vi "SE5082_fieldramp.vi"(6 "Variables":T4=[{"Value"=10.0, "Variable"="dummy", "Save with Image"=FALSE}, {"Value"=-0.0001, "Variable"="HI", "Save with Image"=FALSE}, {"Value"=-0.0002, "Variable"="LO", "Save with Image"=FALSE}, {"Value"=0.0, "Variable"="dummy1", "Save with Image"=FALSE}, {"Value"=0.0, "Variable"="dummy2", "Save with Image"=FALSE}, {"Value"=0.0, "Variable"="dummy3", "Save with Image"=FALSE}, {"Value"=0.0, "Variable"="tLEDuv", "Save with Image"=FALSE}, {"Value"=1000.0, "Variable"="tMOT0", "Save with Image"=FALSE}, {"Value"=20.0, "Variable"="tMOT1", "Save with Image"=FALSE}, {"Value"=40.0, "Variable"="tMOT2", "Save with Image"=FALSE}, {"Value"=50.0, "Variable"="tMOT3", "Save with Image"=FALSE}, {"Value"=13.0, "Variable"="tMOT3delayREP", "Save with Image"=FALSE}, {"Value"=0.05, "Variable"="tREP", "Save with Image"=FALSE}, {"Value"=0.75, "Variable"="dMOT0", "Save with Image"=FALSE}, {"Value"=1.75, "Variable"="dMOT1", "Save with Image"=FALSE}, {"Value"=1.75, "Variable"="dMOT2", "Save with Image"=FALSE}, {"Value"=0.0, "Variable"="dummy5", "Save with Image"=FALSE}, {"Value"=1.45, "Variable"="pMOT0", "Save with Image"=FALSE}, {"Value"=1.45, "Variable"="pMOT1", "Save with Image"=FALSE}, {"Value"=1.25, "Variable"="pMOT2", "Save with Image"=FALSE}, {"Value"=-1.0, "Variable"="dummy6", "Save with Image"=FALSE}, {"Value"=1.6, "Variable"="pRP0", "Save with Image"=FALSE}, {"Value"=1.6, "Variable"="pRP1", "Save with Image"=FALSE}, {"Value"=0.8, "Variable"="pRP2", "Save with Image"=FALSE}, {"Value"=0.0, "Variable"="MOTdummy0", "Save with Image"=FALSE}, {"Value"=-1.0, "Variable"="MOTdummy1", "Save with Image"=FALSE}, {"Value"=0.0, "Variable"="MOTdummy2", "Save with Image"=FALSE}, {"Value"=0.0, "Variable"="MOTdummy3", "Save with Image"=FALSE}, {"Value"=0.0, "Variable"="MOTdummy4", "Save with Image"=FALSE}, {"Value"=1.8, "Variable"="pCROSS0", "Save with Image"=FALSE}, {"Value"=1.29, "Variable"="pCROSS1", "Save with Image"=FALSE}, {"Value"=1.05, "Variable"="pCROSS2", "Save with Image"=FALSE}, {"Value"=0.75, "Variable"="pCROSS3", "Save with Image"=FALSE}, {"Value"=0.0, "Variable"="pCROSS4", "Save with Image"=FALSE}, {"Value"=5.0, "Variable"="pDIMPL0", "Save with Image"=FALSE}, {"Value"=4.4, "Variable"="pDIMPL1", "Save with Image"=FALSE}, {"Value"=3.65, "Variable"="pDIMPL2", "Save with Image"=FALSE}, {"Value"=3.55, "Variable"="pDIMPL3", "Save with Image"=FALSE}, {"Value"=3.45, "Variable"="pDIMPL4", "Save with Image"=FALSE}, {"Value"=1.8, "Variable"="pTightTrap", "Save with Image"=FALSE}, {"Value"=400.0, "Variable"="tHOLD", "Save with Image"=FALSE}, {"Value"=740.0, "Variable"="tEVAP1", "Save with Image"=FALSE}, {"Value"=2900.0, "Variable"="tEVAP2", "Save with Image"=FALSE}, {"Value"=590.0, "Variable"="tEVAP3", "Save with Image"=FALSE}, {"Value"=50.0, "Variable"="tEVAP4", "Save with Image"=FALSE}, {"Value"=50.0, "Variable"="tHOLDTight", "Save with Image"=FALSE}, {"Value"=0.0, "Variable"="ODTdummy1", "Save with Image"=FALSE}, {"Value"=0.0, "Variable"="ODTdummy2", "Save with Image"=FALSE}, {"Value"=0.0, "Variable"="ODTdummy3", "Save with Image"=FALSE}, {"Value"=0.0, "Variable"="ODTdummy4", "Save with Image"=FALSE}, {"Value"=0.0, "Variable"="ODTdummy5", "Save with Image"=FALSE}, {"Value"=3.59, "Variable"="dIMGx", "Save with Image"=FALSE}, {"Value"=3.59, "Variable"="dIMGx0", "Save with Image"=FALSE}, {"Value"=1.38, "Variable"="dIMGz", "Save with Image"=FALSE}, {"Value"=1.98, "Variable"="dEXCz", "Save with Image"=FALSE}, {"Value"=3.0, "Variable"="pABSx", "Save with Image"=FALSE}, {"Value"=1.35, "Variable"="pABSz", "Save with Image"=FALSE}, {"Value"=0.55, "Variable"="pEXCz", "Save with Image"=FALSE}, {"Value"=0.0, "Variable"="TOF", "Save with Image"=FALSE}, {"Value"=10.0, "Variable"="TOFatomFall", "Save with Image"=FALSE}, {"Value"=0.012, "Variable"="tEXP", "Save with Image"=FALSE}, {"Value"=0.2, "Variable"="tEXP2", "Save with Image"=FALSE}, {"Value"=0.082, "Variable"="tEXC", "Save with Image"=FALSE}, {"Value"=0.001, "Variable"="tWaitIoniz", "Save with Image"=FALSE}, {"Value"=0.065, "Variable"="tCAM", "Save with Image"=FALSE}, {"Value"=200.0, "Variable"="tCAMguppy", "Save with Image"=FALSE}, {"Value"=50.0, "Variable"="tCAMreadout", "Save with Image"=FALSE}, {"Value"=-0.002, "Variable"="tTrigDelay", "Save with Image"=FALSE}, {"Value"=0.0, "Variable"="tTrans", "Save with Image"=FALSE}, {"Value"=1.0, "Variable"="tEXCres", "Save with Image"=FALSE}, {"Value"=0.004, "Variable"="tPUMP", "Save with Image"=FALSE}, {"Value"=2.0, "Variable"="pBLUEswitch", "Save with Image"=FALSE}, {"Value"=2.0, "Variable"="pBLUEswitchEIT", "Save with Image"=FALSE}, {"Value"=3.5, "Variable"="dBLUE", "Save with Image"=FALSE}, {"Value"=3.5, "Variable"="dBLUE0", "Save with Image"=FALSE}, {"Value"=1.7, "Variable"="dBLUEdec", "Save with Image"=FALSE}, {"Value"=2.5, "Variable"="dBLUEdec0", "Save with Image"=FALSE}, {"Value"=3.2, "Variable"="dIMPnew", "Save with Image"=FALSE}, {"Value"=1.0, "Variable"="blueON1", "Save with Image"=FALSE}, {"Value"=0.0, "Variable"="blueON2", "Save with Image"=FALSE}, {"Value"=1.0, "Variable"="blueEXCON1", "Save with Image"=FALSE}, {"Value"=0.0, "Variable"="blueEXCON2", "Save with Image"=FALSE}, {"Value"=35.637858, "Variable"="dRydMW", "Save with Image"=FALSE}, {"Value"=16.0, "Variable"="pRydMW", "Save with Image"=FALSE}, {"Value"=50.0, "Variable"="MWduration", "Save with Image"=FALSE}, {"Value"=4.33, "Variable"="bmw0", "Save with Image"=FALSE}, {"Value"=0.02, "Variable"="bmw1", "Save with Image"=FALSE}, {"Value"=0.0, "Variable"="MWdummy1", "Save with Image"=FALSE}, {"Value"=0.0, "Variable"="MWdummy2", "Save with Image"=FALSE}, {"Value"=0.0, "Variable"="MWdummy3", "Save with Image"=FALSE}, {"Value"=4.3, "Variable"="foffset", "Save with Image"=FALSE}, {"Value"=8.64, "Variable"="fdx", "Save with Image"=FALSE}, {"Value"=-5.78, "Variable"="fdy", "Save with Image"=FALSE}, {"Value"=4.0, "Variable"="fdz", "Save with Image"=FALSE}, {"Value"=300.0, "Variable"="CH203", "Save with Image"=FALSE}, {"Value"=160.0, "Variable"="CH215", "Save with Image"=FALSE}, {"Value"=4.0, "Variable"="CH302", "Save with Image"=FALSE}, {"Value"=280.0, "Variable"="CH315", "Save with Image"=FALSE}, {"Value"=0.0, "Variable"="CH202", "Save with Image"=FALSE}, {"Value"=0.0, "Variable"="CH308", "Save with Image"=FALSE}, {"Value"=0.0, "Variable"="EFIELDdummy2", "Save with Image"=FALSE}, {"Value"=0.0, "Variable"="EFIELDdummy3", "Save with Image"=FALSE}, {"Value"=0.0, "Variable"="EFIELDdummy4", "Save with Image"=FALSE}, {"Value"=0.0, "Variable"="EFIELDdummy5", "Save with Image"=FALSE}, {"Value"=0.0, "Variable"="EFIELDdummy6", "Save with Image"=FALSE}, {"Value"=0.0, "Variable"="EFIELDdummy7", "Save with Image"=FALSE}, {"Value"=1.25, "Variable"="bMOT0", "Save with Image"=FALSE}, {"Value"=2.5, "Variable"="bMOT1", "Save with Image"=FALSE}, {"Value"=2.5, "Variable"="bMOT2", "Save with Image"=FALSE}, {"Value"=1.25, "Variable"="bMOT3", "Save with Image"=FALSE}, {"Value"=0.0, "Variable"="bCOMPx", "Save with Image"=FALSE}, {"Value"=1.35, "Variable"="bCOMPy", "Save with Image"=FALSE}, {"Value"=0.27, "Variable"="bCOMPz", "Save with Image"=FALSE}, {"Value"=0.7, "Variable"="bCOMPx1", "Save with Image"=FALSE}, {"Value"=1.1, "Variable"="bCOMPy1", "Save with Image"=FALSE}, {"Value"=0.5, "Variable"="bCOMPz1", "Save with Image"=FALSE}, {"Value"=4.35, "Variable"="bxfinal", "Save with Image"=FALSE}, {"Value"=0.0, "Variable"="byfinal", "Save with Image"=FALSE}, {"Value"=0.0, "Variable"="bzfinal", "Save with Image"=FALSE}, {"Value"=0.0, "Variable"="BFIELDdummy1", "Save with Image"=FALSE}, {"Value"=0.0, "Variable"="BFIELDdummy2", "Save with Image"=FALSE}, {"Value"=0.0, "Variable"="BFIELDdummy3", "Save with Image"=FALSE}, {"Value"=10.0, "Variable"="tCOILsettle", "Save with Image"=FALSE}, {"Value"=0.0, "Variable"="tRemove", "Save with Image"=FALSE}, {"Value"=3.6, "Variable"="pRemove", "Save with Image"=FALSE}, {"Value"=3.1, "Variable"="dF2CLEAN1x", "Save with Image"=FALSE}, {"Value"=20.0, "Variable"="tF2CLEAN1x", "Save with Image"=FALSE}, {"Value"=4.0, "Variable"="tF2CLEAN2x", "Save with Image"=FALSE}, {"Value"=0.0, "Variable"="tDelayDown", "Save with Image"=FALSE}, {"Value"=156.0, "Variable"="oDDSbluePro", "Save with Image"=FALSE}, {"Value"=-10.25, "Variable"="dDDSbluePro", "Save with Image"=FALSE}, {"Value"=50.0, "Variable"="tRampDDSbluePro", "Save with Image"=FALSE}, {"Value"=416.6261, "Variable"="oDDSred", "Save with Image"=FALSE}, {"Value"=-50.25, "Variable"="dDDSred", "Save with Image"=FALSE}, {"Value"=90.0, "Variable"="tRampDDSred", "Save with Image"=FALSE}, {"Value"=154.0, "Variable"="oDDSblueOld", "Save with Image"=FALSE}, {"Value"=10.0, "Variable"="dDDSblueOld", "Save with Image"=FALSE}, {"Value"=100.0, "Variable"="tRampDDSblueOld", "Save with Image"=FALSE}, {"Value"=1.0, "Variable"="mwON", "Save with Image"=FALSE}, {"Value"=9.4e-05, "Variable"="tRabi", "Save with Image"=FALSE}, {"Value"=9.4e-05, "Variable"="tRabi2", "Save with Image"=FALSE}, {"Value"=5e-05, "Variable"="tRamsey", "Save with Image"=FALSE}, {"Value"=0.0, "Variable"="tRamsey2", "Save with Image"=FALSE}, {"Value"=0.0, "Variable"="tDDSa", "Save with Image"=FALSE}, {"Value"=0.0, "Variable"="tDDSb", "Save with Image"=FALSE}, {"Value"=399.942, "Variable"="dDDSa", "Save with Image"=FALSE}, {"Value"=399.942, "Variable"="dDDSa2", "Save with Image"=FALSE}, {"Value"=0.2, "Variable"="pDDSa", "Save with Image"=FALSE}, {"Value"=1e-07, "Variable"="pDDSa2", "Save with Image"=FALSE}, {"Value"=0.0, "Variable"="phiDDSa", "Save with Image"=FALSE}, {"Value"=0.875, "Variable"="phiDDSa2", "Save with Image"=FALSE}, {"Value"=399.942, "Variable"="dDDSb", "Save with Image"=FALSE}, {"Value"=400.009, "Variable"="dDDSb2", "Save with Image"=FALSE}, {"Value"=0.25, "Variable"="pDDSb", "Save with Image"=FALSE}, {"Value"=1e-07, "Variable"="pDDSb2", "Save with Image"=FALSE}, {"Value"=0.25, "Variable"="phiDDSb", "Save with Image"=FALSE}, {"Value"=0.55, "Variable"="phiDDSb2", "Save with Image"=FALSE}, {"Value"=300.0, "Variable"="tDipole", "Save with Image"=FALSE}, {"Value"=0.7, "Variable"="bCOMPx2", "Save with Image"=FALSE}, {"Value"=0.8, "Variable"="bCOMPy2", "Save with Image"=FALSE}, {"Value"=0.6, "Variable"="bCOMPz2", "Save with Image"=FALSE}, {"Value"=20.0, "Variable"="dMOTRamp1", "Save with Image"=FALSE}, {"Value"=18.0, "Variable"="DMOTload", "Save with Image"=FALSE}, {"Value"=50.0, "Variable"="dMOTRamp2", "Save with Image"=FALSE}, {"Value"=272.0, "Variable"="DMOTimag", "Save with Image"=FALSE}, {"Value"=1000.0, "Variable"="oDDShyperfine", "Save with Image"=FALSE}, {"Value"=0.1, "Variable"="dDDShyperfine", "Save with Image"=FALSE}, {"Value"=0.0, "Variable"="tof", "Save with Image"=FALSE}, {"Value"=262.5, "Variable"="dOPump", "Save with Image"=FALSE}, {"Value"=4500.0, "Variable"="tRampOPump", "Save with Image"=FALSE}, {"Value"=10.0, "Variable"="tOPump", "Save with Image"=FALSE}, {"Value"=1.5, "Variable"="bCOMPx3", "Save with Image"=FALSE}, {"Value"=0.8, "Variable"="bCOMPy3", "Save with Image"=FALSE}, {"Value"=0.0, "Variable"="bCOMPz3", "Save with Image"=FALSE}, {"Value"=0.0, "Variable"="bCOMPx4", "Save with Image"=FALSE}, {"Value"=0.0, "Variable"="bCOMPy4", "Save with Image"=FALSE}, {"Value"=0.0, "Variable"="bCOMPz4", "Save with Image"=FALSE}, {"Value"=0.0, "Variable"="scan2photRes", "Save with Image"=FALSE}, {"Value"=0.0, "Variable"="tEXCsmallProbe", "Save with Image"=FALSE}, {"Value"=0.082, "Variable"="tEXCBlue", "Save with Image"=FALSE}, {"Value"=0.0015, "Variable"="tDownPump", "Save with Image"=FALSE}, {"Value"=98.75, "Variable"="RF1freq1", "Save with Image"=FALSE}, {"Value"=0.1, "Variable"="RF1freq2", "Save with Image"=FALSE}, {"Value"=98.75, "Variable"="dummya", "Save with Image"=FALSE}, {"Value"=0.1, "Variable"="dummyb", "Save with Image"=FALSE}] {"Value" format="%#.9g"}, 8 "error in (no error)":errorcluster, 10 "HV_variables":T3={"Sampling rate"=50000000, "Amplifier gain"=-100.0, "Waveform"=[{"waveform"=1, "duration"="1", "e-factor"="-5", "Vinit"="0", "Vfinal"="1"}, {"waveform"=0, "duration"="1", "e-factor"="0", "Vinit"="1", "Vfinal"="1"}, {"waveform"=0, "duration"="1", "e-factor"="-5", "Vinit"="1", "Vfinal"="0"}], "Load waveform"=TRUE, "CH1_LO"="0", "CH1_HI"="400", "CH2_LO"="0", "CH2_HI"="-100"} {"Sampling rate" format="%.0p"; "Waveform"."waveform" items=["Linear Ramp", "Exp Rise", "Exp Decay"]}, 11 "VISA resource name in":refnum<visa-resource-name>="TCPIP0::10.11.1.75::inst0::INSTR") -> (0 "error out":errorcluster={"status"=TRUE, "code"=-1073807194, "source"="VISA Write in DG1022z_fieldramp.vi->HV_Amplifier_out.vi"}, 1 "Output to electrodes2":cluster{dbl[], "y":dbl[]}(graph)={[0.0, 0.02, 0.04, 0.06, 0.08, 0.09999999999999999, 0.12, 0.14, 0.16, 0.18, 0.19999999999999998, 0.22, 0.24, 0.26, 0.28, 0.3, 0.32, 0.33999999999999997, 0.36, 0.38, 0.39999999999999997, 0.42, 0.44, 0.45999999999999996, 0.48, 0.5, 0.52, 0.54, 0.56, 0.58, 0.6, 0.62, 0.64, 0.66, 0.6799999999999999, 0.7, 0.72, 0.74, 0.76, 0.78, 0.7999999999999999, 0.82, 0.84, 0.86, 0.88, 0.8999999999999999, 0.9199999999999999, 0.94, 0.96, 0.98, 1.0, 1.02, 1.04, 1.06, 1.08, 1.1, 1.1199999999999999, 1.14, 1.16, 1.18, 1.2, 1.22, 1.24, 1.26, 1.28, 1.2999999999999998, 1.32, 1.3399999999999999, 1.3599999999999999, 1.38, 1.4, 1.42, 1.44, 1.46, 1.4799999999999998, 1.5, 1.5199999999999998, 1.54, 1.5599999999999998, 1.5799999999999998, 1.5999999999999999, 1.6199999999999999, 1.64, 1.66, 1.68, 1.6999999999999997, 1.72, 1.7399999999999998, 1.76, 1.7799999999999998, 1.7999999999999998, 1.8199999999999998, 1.8399999999999999, 1.8599999999999999, 1.88, 1.9, 1.92, 1.9400000000000002, 1.96, 1.9799999999999998, 2.0, 2.0199999999999996, 2.04, 2.0599999999999996, 2.08, 2.0999999999999996, 2.12, 2.1399999999999997, 2.16, 2.1799999999999997, 2.2, 2.2199999999999998, 2.2399999999999998, 2.26, 2.28, 2.3, 2.32, 2.34, 2.36, 2.38, 2.4, 2.4199999999999995, 2.44, 2.4599999999999995, 2.48, 2.5, 2.52, 2.54, 2.56, 2.58, 2.5999999999999996, 2.62, 2.64, 2.66, 2.6799999999999997, 2.7, 2.7199999999999998, 2.74, 2.76, 2.7800000000000002, 2.8, 2.8200000000000003, 2.84, 2.86, 2.88, 2.9, 2.92, 2.94, 2.9599999999999995, 2.98, 3.0], "y"=[0.0, -9.580813208007743, -18.249891493826283, -26.093997906717924, -33.19163890015812, -39.61385005080873, -45.424907006445174, -50.682968778243165, -55.44065981571043, -59.745596689865145, -63.64086465588308, -67.16544886481294, -70.35462454007137, -73.24031002373526, -75.85138622603756, -78.21398567522392, -80.35175406067887, -82.28608688693284, -84.03634360706266, -85.62004137860504, -87.05303038115674, -88.34965245029956, -89.52288461551117, -90.584468978638, -91.54503023279702, -92.41418199787564, -93.2006230368708, -93.91222431603269, -94.55610778014061, -95.13871763132006, -95.66588482478362, -96.14288542699043, -96.57449342029285, -96.96502848255628, -97.31839921994724, -97.63814228557754, -97.92745777551737, -98.18924125643233, -98.42611274538788, -98.64044293186076, -98.83437690439604, -99.00985561937433, -99.16863532675555, -99.31230514721888, -99.4423029766166, -99.55992987691913, -99.66636309768043, -99.76266785834734, -99.84980800933376, -99.92865567855956, -100.0, -100.0, -100.0, -100.0, -100.0, -100.0, -100.0, -100.0, -100.0, -100.0, -100.0, -100.0, -100.0, -100.0, -100.0, -100.0, -100.0, -100.0, -100.0, -100.0, -100.0, -100.0, -100.0, -100.0, -100.0, -100.0, -100.0, -100.0, -100.0, -100.0, -100.0, -100.0, -100.0, -100.0, -100.0, -100.0, -100.0, -100.0, -100.0, -100.0, -100.0, -100.0, -100.0, -100.0, -100.0, -100.0, -100.0, -100.0, -100.0, -100.0, -100.0, -98.0, -96.0, -94.0, -92.0, -90.0, -88.0, -86.0, -84.0, -82.0, -80.0, -78.0, -76.0, -74.0, -72.0, -70.0, -68.0, -65.99999999999999, -64.0, -62.0, -60.0, -58.00000000000001, -56.00000000000001, -54.0, -52.0, -50.0, -48.0, -46.0, -43.99999999999999, -42.00000000000001, -40.0, -38.0, -36.0, -34.0, -31.999999999999996, -29.999999999999993, -28.000000000000004, -26.0, -24.0, -21.999999999999996, -19.999999999999996, -17.999999999999993, -16.000000000000004, -14.000000000000002, -12.0, -9.999999999999998, -7.9999999999999964, -5.999999999999995, -4.0000000000000036, -2.0000000000000018, 0.0]}, 2 "Output to electrodes1":cluster{dbl[], "y":dbl[]}(graph)={[0.0, 0.02, 0.04, 0.06, 0.08, 0.09999999999999999, 0.12, 0.14, 0.16, 0.18, 0.19999999999999998, 0.22, 0.24, 0.26, 0.28, 0.3, 0.32, 0.33999999999999997, 0.36, 0.38, 0.39999999999999997, 0.42, 0.44, 0.45999999999999996, 0.48, 0.5, 0.52, 0.54, 0.56, 0.58, 0.6, 0.62, 0.64, 0.66, 0.6799999999999999, 0.7, 0.72, 0.74, 0.76, 0.78, 0.7999999999999999, 0.82, 0.84, 0.86, 0.88, 0.8999999999999999, 0.9199999999999999, 0.94, 0.96, 0.98, 1.0, 1.02, 1.04, 1.06, 1.08, 1.1, 1.1199999999999999, 1.14, 1.16, 1.18, 1.2, 1.22, 1.24, 1.26, 1.28, 1.2999999999999998, 1.32, 1.3399999999999999, 1.3599999999999999, 1.38, 1.4, 1.42, 1.44, 1.46, 1.4799999999999998, 1.5, 1.5199999999999998, 1.54, 1.5599999999999998, 1.5799999999999998, 1.5999999999999999, 1.6199999999999999, 1.64, 1.66, 1.68, 1.6999999999999997, 1.72, 1.7399999999999998, 1.76, 1.7799999999999998, 1.7999999999999998, 1.8199999999999998, 1.8399999999999999, 1.8599999999999999, 1.88, 1.9, 1.92, 1.9400000000000002, 1.96, 1.9799999999999998, 2.0, 2.0199999999999996, 2.04, 2.0599999999999996, 2.08, 2.0999999999999996, 2.12, 2.1399999999999997, 2.16, 2.1799999999999997, 2.2, 2.2199999999999998, 2.2399999999999998, 2.26, 2.28, 2.3, 2.32, 2.34, 2.36, 2.38, 2.4, 2.4199999999999995, 2.44, 2.4599999999999995, 2.48, 2.5, 2.52, 2.54, 2.56, 2.58, 2.5999999999999996, 2.62, 2.64, 2.66, 2.6799999999999997, 2.7, 2.7199999999999998, 2.74, 2.76, 2.7800000000000002, 2.8, 2.8200000000000003, 2.84, 2.86, 2.88, 2.9, 2.92, 2.94, 2.9599999999999995, 2.98, 3.0], "y"=[0.0, -9.580813208007743, -18.249891493826283, -26.093997906717924, -33.19163890015812, -39.61385005080873, -45.424907006445174, -50.682968778243165, -55.44065981571043, -59.745596689865145, -63.64086465588308, -67.16544886481294, -70.35462454007137, -73.24031002373526, -75.85138622603756, -78.21398567522392, -80.35175406067887, -82.28608688693284, -84.03634360706266, -85.62004137860504, -87.05303038115674, -88.34965245029956, -89.52288461551117, -90.584468978638, -91.54503023279702, -92.41418199787564, -93.2006230368708, -93.91222431603269, -94.55610778014061, -95.13871763132006, -95.66588482478362, -96.14288542699043, -96.57449342029285, -96.96502848255628, -97.31839921994724, -97.63814228557754, -97.92745777551737, -98.18924125643233, -98.42611274538788, -98.64044293186076, -98.83437690439604, -99.00985561937433, -99.16863532675555, -99.31230514721888, -99.4423029766166, -99.55992987691913, -99.66636309768043, -99.76266785834734, -99.84980800933376, -99.92865567855956, -100.0, -100.0, -100.0, -100.0, -100.0, -100.0, -100.0, -100.0, -100.0, -100.0, -100.0, -100.0, -100.0, -100.0, -100.0, -100.0, -100.0, -100.0, -100.0, -100.0, -100.0, -100.0, -100.0, -100.0, -100.0, -100.0, -100.0, -100.0, -100.0, -100.0, -100.0, -100.0, -100.0, -100.0, -100.0, -100.0, -100.0, -100.0, -100.0, -100.0, -100.0, -100.0, -100.0, -100.0, -100.0, -100.0, -100.0, -100.0, -100.0, -100.0, -100.0, -98.0, -96.0, -94.0, -92.0, -90.0, -88.0, -86.0, -84.0, -82.0, -80.0, -78.0, -76.0, -74.0, -72.0, -70.0, -68.0, -65.99999999999999, -64.0, -62.0, -60.0, -58.00000000000001, -56.00000000000001, -54.0, -52.0, -50.0, -48.0, -46.0, -43.99999999999999, -42.00000000000001, -40.0, -38.0, -36.0, -34.0, -31.999999999999996, -29.999999999999993, -28.000000000000004, -26.0, -24.0, -21.999999999999996, -19.999999999999996, -17.999999999999993, -16.000000000000004, -14.000000000000002, -12.0, -9.999999999999998, -7.9999999999999964, -5.999999999999995, -4.0000000000000036, -2.0000000000000018, 0.0]}, 3 "VISA resource name out":refnum<visa-resource-name>="TCPIP0::10.11.1.75::inst0::INSTR")   [LabVIEW 2017]
uses:
  Software/Rydberg_Control/TypeDefinition/variables.ctl
  sequence_variables.ctl
panel:
  in  "Save sequence":bool
  in  "AWG sequence_variables":T1={"Sampling rate"=50000000, "Waveform"=[{"segment number"="1", "repeat"="-5", "jump flag"="0", "segment name"=0}, {"segment number"="1", "repeat"="0", "jump flag"="1", "segment name"=0}, {"segment number"="1", "repeat"="-5", "jump flag"="1", "segment name"=0}], "Load waveform"=FALSE, "CH1_LO"="0", "CH1_HI"="300", "CH2_LO"="0", "CH2_HI"="300"} {"Sampling rate" format="%.0p"; "Waveform"."segment name" items=["Linear Ramp", "Exp Rise", "Exp Decay"]}
  in  "Array":bool[](array[boolean])=[FALSE, TRUE]
  in  "waveform name":string[](array[string])=["000.RAF", "001.RAF"]
  in  "Debug array 2":string[](array[string])=["*CLS\n", "*RST\n", ":SOUR1:APPL:ARB 50E6,10,0", ":SOUR1:DATA VOLATILE,-0.000000,-0.049101,-0.095808,-0.140237,-0.182499,-0.222700,-0.260940,-0.297315,-0.331916,-0.364830,-0.396139,-0.425920,-0.454249,-0.481196,-0.506830,-0.531213,-0.554407,-0.576469,-0.597456,-0.617419,-0.636409,-0.654472,-0.671654,-0.687999,-0.703546,-0.718335,-0.732403,-0.745785,-0.758514,-0.770622,-0.782140,-0.793096,-0.803518,-0.813431,-0.822861,-0.831831,-0.840363,-0.848480,-0.856200,-0.863544,-0.870530,-0.877175,-0.883497,-0.889509,-0.895229,-0.900669,-0.905845,-0.910768,-0.915450,-0.919905,-0.924142,-0.928172,-0.932006,-0.935653,-0.939122,-0.942422,-0.945561,-0.948547,-0.951387,-0.954089,-0.956659,-0.959103,-0.961429,-0.963641,-0.965745,-0.967746,-0.969650,-0.971461,-0.973184,-0.974823,-0.976381,-0.977864,-0.979275,-0.980616,-0.981892,-0.983106,-0.984261,-0.985360,-0.986404,-0.987398,-0.988344,-0.989243,-0.990099,-0.990912,-0.991686,-0.992423,-0.993123,-0.993789,-0.994423,-0.995026,-0.995599,-0.996145,-0.996664,-0.997157,-0.997627,-0.998073,-0.998498,-0.998902,-0.999287,-0.999652,-1.000000,-1.000000,-1.000000,-1.000000,-1.000000,-1.000000,-1.000000,-1.000000,-1.000000,-1.000000,-1.000000,-1.000000,-1.000000,-1.000000,-1.000000,-1.000000,-1.000000,-1.000000,-1.000000,-1.000000,-1.000000,-1.000000,-1.000000,-1.000000,-1.000000,-1.000000,-1.000000,-1.000000,-1.000000,-1.000000,-1.000000,-1.000000,-1.000000,-1.000000,-1.000000,-1.000000,-1.000000,-1.000000,-1.000000,-1.000000,-1.000000,-1.000000,-1.000000,-1.000000,-1.000000,-1.000000,-1.000000,-1.000000,-1.000000,-1.000000,-1.000000,-0.980000,-0.960000,-0.940000,-0.920000,-0.900000,-0.880000,-0.860000,-0.840000,-0.820000,-0.800000,-0.780000,-0.760000,-0.740000,-0.720000,-0.700000,-0.680000,-0.660000,-0.640000,-0.620000,-0.600000,-0.580000,-0.560000,-0.540000,-0.520000,-0.500000,-0.480000,-0.460000,-0.440000,-0.420000,-0.400000,-0.380000,-0.360000,-0.340000,-0.320000,-0.300000,-0.280000,-0.260000,-0.240000,-0.220000,-0.200000,-0.180000,-0.160000,-0.140000,-0.120000,-0.100000,-0.080000,-0.060000,-0.040000,-0.020000,-0.000000", ":SOUR1:BURS:STAT ON", ":SOUR1:BURS:MODE TRIG", ":SOUR1:BURS:NCYC 1", ":SOUR1:BURS:TRIG:SOUR EXT", ":SOUR1:BURS ON", ":SOUR1:BURSt:IDLE FPT", ":OUTP:LOAD INF", ":OUTP1 ON"]
  in  "waveform name 2":string="000.RAF"
  out "Input waveform commands 2":string[](array[string])=["*CLS", "*RST", ":SOUR1:APPL:ARB 50000000", ":SOUR1:DATA VOLATILE,-0.000000,0.095808,0.182499,0.260940,0.331916,0.396139,0.454249,0.506830,0.554407,0.597456,0.636409,0.671654,0.703546,0.732403,0.758514,0.782140,0.803518,0.822861,0.840363,0.856200,0.870530,0.883497,0.895229,0.905845,0.915450,0.924142,0.932006,0.939122,0.945561,0.951387,0.956659,0.961429,0.965745,0.969650,0.973184,0.976381,0.979275,0.981892,0.984261,0.986404,0.988344,0.990099,0.991686,0.993123,0.994423,0.995599,0.996664,0.997627,0.998498,0.999287,1.000000,1.000000,1.000000,1.000000,1.000000,1.000000,1.000000,1.000000,1.000000,1.000000,1.000000,1.000000,1.000000,1.000000,1.000000,1.000000,1.000000,1.000000,1.000000,1.000000,1.000000,1.000000,1.000000,1.000000,1.000000,1.000000,1.000000,1.000000,1.000000,1.000000,1.000000,1.000000,1.000000,1.000000,1.000000,1.000000,1.000000,1.000000,1.000000,1.000000,1.000000,1.000000,1.000000,1.000000,1.000000,1.000000,1.000000,1.000000,1.000000,1.000000,1.000000,0.980000,0.960000,0.940000,0.920000,0.900000,0.880000,0.860000,0.840000,0.820000,0.800000,0.780000,0.760000,0.740000,0.720000,0.700000,0.680000,0.660000,0.640000,0.620000,0.600000,0.580000,0.560000,0.540000,0.520000,0.500000,0.480000,0.460000,0.440000,0.420000,0.400000,0.380000,0.360000,0.340000,0.320000,0.300000,0.280000,0.260000,0.240000,0.220000,0.200000,0.180000,0.160000,0.140000,0.120000,0.100000,0.080000,0.060000,0.040000,0.020000,-0.000000", ":SOUR1:DATA:COPY 000.RAF, VOLATILE", ":SOUR1:FUNC USER 000.RAF", ":SOUR1:BURS:STAT ON", ":SOUR1:BURS:MODE TRIG", ":SOUR1:BURS:NCYC 1", ":SOUR1:BURS:TRIG:SOUR EXT", ":SOUR1:BURS ON", ":SOUR1:BURSt:IDLE FPT", ":OUTP:LOAD INF"]
  out "waveform to CH2":dbl[](array[numeric])=[-0.0, 0.09580813208007743, 0.18249891493826284, 0.26093997906717925, 0.33191638900158116, 0.3961385005080873, 0.45424907006445175, 0.5068296877824316, 0.5544065981571044, 0.5974559668986514, 0.6364086465588308, 0.6716544886481295, 0.7035462454007138, 0.7324031002373527, 0.7585138622603756, 0.7821398567522393, 0.8035175406067887, 0.8228608688693284, 0.8403634360706266, 0.8562004137860504, 0.8705303038115675, 0.8834965245029955, 0.8952288461551118, 0.90584468978638, 0.9154503023279702, 0.9241418199787564, 0.932006230368708, 0.9391222431603269, 0.9455610778014061, 0.9513871763132006, 0.9566588482478362, 0.9614288542699043, 0.9657449342029285, 0.9696502848255628, 0.9731839921994724, 0.9763814228557754, 0.9792745777551737, 0.9818924125643232, 0.9842611274538788, 0.9864044293186076, 0.9883437690439604, 0.9900985561937433, 0.9916863532675555, 0.9931230514721888, 0.994423029766166, 0.9955992987691913, 0.9966636309768043, 0.9976266785834734, 0.9984980800933375, 0.9992865567855956, 1.0, 1.0, 1.0, 1.0, 1.0, 1.0, 1.0, 1.0, 1.0, 1.0, 1.0, 1.0, 1.0, 1.0, 1.0, 1.0, 1.0, 1.0, 1.0, 1.0, 1.0, 1.0, 1.0, 1.0, 1.0, 1.0, 1.0, 1.0, 1.0, 1.0, 1.0, 1.0, 1.0, 1.0, 1.0, 1.0, 1.0, 1.0, 1.0, 1.0, 1.0, 1.0, 1.0, 1.0, 1.0, 1.0, 1.0, 1.0, 1.0, 1.0, 1.0, 0.98, 0.96, 0.94, 0.92, 0.9, 0.88, 0.86, 0.84, 0.82, 0.8, 0.78, 0.76, 0.74, 0.72, 0.7, 0.68, 0.6599999999999998, 0.64, 0.62, 0.6, 0.5800000000000001, 0.56, 0.54, 0.52, 0.5, 0.48, 0.46, 0.43999999999999995, 0.4200000000000001, 0.4, 0.38, 0.36, 0.34, 0.31999999999999995, 0.29999999999999993, 0.28, 0.26, 0.24, 0.21999999999999997, 0.19999999999999996, 0.17999999999999994, 0.16000000000000003, 0.14, 0.12, 0.09999999999999998, 0.07999999999999996, 0.05999999999999995, 0.040000000000000036, 0.020000000000000018, -0.0]
  out "Output to CH2":dbl[](graph)=[-0.0, 0.09580813208007743, 0.18249891493826284, 0.26093997906717925, 0.33191638900158116, 0.3961385005080873, 0.45424907006445175, 0.5068296877824316, 0.5544065981571044, 0.5974559668986514, 0.6364086465588308, 0.6716544886481295, 0.7035462454007138, 0.7324031002373527, 0.7585138622603756, 0.7821398567522393, 0.8035175406067887, 0.8228608688693284, 0.8403634360706266, 0.8562004137860504, 0.8705303038115675, 0.8834965245029955, 0.8952288461551118, 0.90584468978638, 0.9154503023279702, 0.9241418199787564, 0.932006230368708, 0.9391222431603269, 0.9455610778014061, 0.9513871763132006, 0.9566588482478362, 0.9614288542699043, 0.9657449342029285, 0.9696502848255628, 0.9731839921994724, 0.9763814228557754, 0.9792745777551737, 0.9818924125643232, 0.9842611274538788, 0.9864044293186076, 0.9883437690439604, 0.9900985561937433, 0.9916863532675555, 0.9931230514721888, 0.994423029766166, 0.9955992987691913, 0.9966636309768043, 0.9976266785834734, 0.9984980800933375, 0.9992865567855956, 1.0, 1.0, 1.0, 1.0, 1.0, 1.0, 1.0, 1.0, 1.0, 1.0, 1.0, 1.0, 1.0, 1.0, 1.0, 1.0, 1.0, 1.0, 1.0, 1.0, 1.0, 1.0, 1.0, 1.0, 1.0, 1.0, 1.0, 1.0, 1.0, 1.0, 1.0, 1.0, 1.0, 1.0, 1.0, 1.0, 1.0, 1.0, 1.0, 1.0, 1.0, 1.0, 1.0, 1.0, 1.0, 1.0, 1.0, 1.0, 1.0, 1.0, 1.0, 0.98, 0.96, 0.94, 0.92, 0.9, 0.88, 0.86, 0.84, 0.82, 0.8, 0.78, 0.76, 0.74, 0.72, 0.7, 0.68, 0.6599999999999998, 0.64, 0.62, 0.6, 0.5800000000000001, 0.56, 0.54, 0.52, 0.5, 0.48, 0.46, 0.43999999999999995, 0.4200000000000001, 0.4, 0.38, 0.36, 0.34, 0.31999999999999995, 0.29999999999999993, 0.28, 0.26, 0.24, 0.21999999999999997, 0.19999999999999996, 0.17999999999999994, 0.16000000000000003, 0.14, 0.12, 0.09999999999999998, 0.07999999999999996, 0.05999999999999995, 0.040000000000000036, 0.020000000000000018, -0.0]
  out "hvhi2":dbl
  out "hvlo2":dbl
  out "CH2_LO":string="0"
  out "CH2_HI":string="-100"
  out "hvlo1":dbl
  out "hvhi1":dbl
  in  "Readout status?":bool
  out "Load waveform":bool=TRUE
  out "Amplifier gain":dbl=-100.0
  out "CH1_HI":string="-100"
  out "CH1_LO":string="0"
  out "Sampling rate":i32=50000000 format="%.0p"
  out "Waveform":T2(array[cluster])=[{"waveform"=1, "duration"="1", "e-factor"="-5", "Vinit"="0", "Vfinal"="1"}, {"waveform"=0, "duration"="1", "e-factor"="0", "Vinit"="1", "Vfinal"="1"}, {"waveform"=0, "duration"="1", "e-factor"="-5", "Vinit"="1", "Vfinal"="0"}]
  out "Input waveform commands":string[](array[string])=["*CLS", "*RST", ":SOUR1:APPL:ARB 50000000", ":SOUR1:DATA VOLATILE,-0.000000,0.095808,0.182499,0.260940,0.331916,0.396139,0.454249,0.506830,0.554407,0.597456,0.636409,0.671654,0.703546,0.732403,0.758514,0.782140,0.803518,0.822861,0.840363,0.856200,0.870530,0.883497,0.895229,0.905845,0.915450,0.924142,0.932006,0.939122,0.945561,0.951387,0.956659,0.961429,0.965745,0.969650,0.973184,0.976381,0.979275,0.981892,0.984261,0.986404,0.988344,0.990099,0.991686,0.993123,0.994423,0.995599,0.996664,0.997627,0.998498,0.999287,1.000000,1.000000,1.000000,1.000000,1.000000,1.000000,1.000000,1.000000,1.000000,1.000000,1.000000,1.000000,1.000000,1.000000,1.000000,1.000000,1.000000,1.000000,1.000000,1.000000,1.000000,1.000000,1.000000,1.000000,1.000000,1.000000,1.000000,1.000000,1.000000,1.000000,1.000000,1.000000,1.000000,1.000000,1.000000,1.000000,1.000000,1.000000,1.000000,1.000000,1.000000,1.000000,1.000000,1.000000,1.000000,1.000000,1.000000,1.000000,1.000000,1.000000,1.000000,0.980000,0.960000,0.940000,0.920000,0.900000,0.880000,0.860000,0.840000,0.820000,0.800000,0.780000,0.760000,0.740000,0.720000,0.700000,0.680000,0.660000,0.640000,0.620000,0.600000,0.580000,0.560000,0.540000,0.520000,0.500000,0.480000,0.460000,0.440000,0.420000,0.400000,0.380000,0.360000,0.340000,0.320000,0.300000,0.280000,0.260000,0.240000,0.220000,0.200000,0.180000,0.160000,0.140000,0.120000,0.100000,0.080000,0.060000,0.040000,0.020000,-0.000000", ":SOUR1:DATA:COPY 000.RAF, VOLATILE", ":SOUR1:FUNC USER 000.RAF", ":SOUR1:BURS:STAT ON", ":SOUR1:BURS:MODE TRIG", ":SOUR1:BURS:NCYC 1", ":SOUR1:BURS:TRIG:SOUR EXT", ":SOUR1:BURS ON", ":SOUR1:BURSt:IDLE FPT", ":OUTP:LOAD INF"]
  in  "Read-out commands":string[](array[string])=["*IDN?", ":SOUR1:APPL?", ":SOUR1:BURS:STAT?", ":SOUR1:BURS:TRIG:SOUR?", ":OUTP1:LOAD?", ":SOUR2:APPL?", ":SOUR2:BURS:STAT?", ":SOUR2:BURS:TRIG:SOUR?", ":OUTP2:LOAD?", ":SOUR2:FUNC?"]
  out "Output to CH1":dbl[](graph)=[-0.0, 0.09580813208007743, 0.18249891493826284, 0.26093997906717925, 0.33191638900158116, 0.3961385005080873, 0.45424907006445175, 0.5068296877824316, 0.5544065981571044, 0.5974559668986514, 0.6364086465588308, 0.6716544886481295, 0.7035462454007138, 0.7324031002373527, 0.7585138622603756, 0.7821398567522393, 0.8035175406067887, 0.8228608688693284, 0.8403634360706266, 0.8562004137860504, 0.8705303038115675, 0.8834965245029955, 0.8952288461551118, 0.90584468978638, 0.9154503023279702, 0.9241418199787564, 0.932006230368708, 0.9391222431603269, 0.9455610778014061, 0.9513871763132006, 0.9566588482478362, 0.9614288542699043, 0.9657449342029285, 0.9696502848255628, 0.9731839921994724, 0.9763814228557754, 0.9792745777551737, 0.9818924125643232, 0.9842611274538788, 0.9864044293186076, 0.9883437690439604, 0.9900985561937433, 0.9916863532675555, 0.9931230514721888, 0.994423029766166, 0.9955992987691913, 0.9966636309768043, 0.9976266785834734, 0.9984980800933375, 0.9992865567855956, 1.0, 1.0, 1.0, 1.0, 1.0, 1.0, 1.0, 1.0, 1.0, 1.0, 1.0, 1.0, 1.0, 1.0, 1.0, 1.0, 1.0, 1.0, 1.0, 1.0, 1.0, 1.0, 1.0, 1.0, 1.0, 1.0, 1.0, 1.0, 1.0, 1.0, 1.0, 1.0, 1.0, 1.0, 1.0, 1.0, 1.0, 1.0, 1.0, 1.0, 1.0, 1.0, 1.0, 1.0, 1.0, 1.0, 1.0, 1.0, 1.0, 1.0, 1.0, 0.98, 0.96, 0.94, 0.92, 0.9, 0.88, 0.86, 0.84, 0.82, 0.8, 0.78, 0.76, 0.74, 0.72, 0.7, 0.68, 0.6599999999999998, 0.64, 0.62, 0.6, 0.5800000000000001, 0.56, 0.54, 0.52, 0.5, 0.48, 0.46, 0.43999999999999995, 0.4200000000000001, 0.4, 0.38, 0.36, 0.34, 0.31999999999999995, 0.29999999999999993, 0.28, 0.26, 0.24, 0.21999999999999997, 0.19999999999999996, 0.17999999999999994, 0.16000000000000003, 0.14, 0.12, 0.09999999999999998, 0.07999999999999996, 0.05999999999999995, 0.040000000000000036, 0.020000000000000018, -0.0]
  out "Status output":string[](array[string])
  out "waveform to CH1":dbl[](array[numeric])=[-0.0, 0.09580813208007743, 0.18249891493826284, 0.26093997906717925, 0.33191638900158116, 0.3961385005080873, 0.45424907006445175, 0.5068296877824316, 0.5544065981571044, 0.5974559668986514, 0.6364086465588308, 0.6716544886481295, 0.7035462454007138, 0.7324031002373527, 0.7585138622603756, 0.7821398567522393, 0.8035175406067887, 0.8228608688693284, 0.8403634360706266, 0.8562004137860504, 0.8705303038115675, 0.8834965245029955, 0.8952288461551118, 0.90584468978638, 0.9154503023279702, 0.9241418199787564, 0.932006230368708, 0.9391222431603269, 0.9455610778014061, 0.9513871763132006, 0.9566588482478362, 0.9614288542699043, 0.9657449342029285, 0.9696502848255628, 0.9731839921994724, 0.9763814228557754, 0.9792745777551737, 0.9818924125643232, 0.9842611274538788, 0.9864044293186076, 0.9883437690439604, 0.9900985561937433, 0.9916863532675555, 0.9931230514721888, 0.994423029766166, 0.9955992987691913, 0.9966636309768043, 0.9976266785834734, 0.9984980800933375, 0.9992865567855956, 1.0, 1.0, 1.0, 1.0, 1.0, 1.0, 1.0, 1.0, 1.0, 1.0, 1.0, 1.0, 1.0, 1.0, 1.0, 1.0, 1.0, 1.0, 1.0, 1.0, 1.0, 1.0, 1.0, 1.0, 1.0, 1.0, 1.0, 1.0, 1.0, 1.0, 1.0, 1.0, 1.0, 1.0, 1.0, 1.0, 1.0, 1.0, 1.0, 1.0, 1.0, 1.0, 1.0, 1.0, 1.0, 1.0, 1.0, 1.0, 1.0, 1.0, 1.0, 0.98, 0.96, 0.94, 0.92, 0.9, 0.88, 0.86, 0.84, 0.82, 0.8, 0.78, 0.76, 0.74, 0.72, 0.7, 0.68, 0.6599999999999998, 0.64, 0.62, 0.6, 0.5800000000000001, 0.56, 0.54, 0.52, 0.5, 0.48, 0.46, 0.43999999999999995, 0.4200000000000001, 0.4, 0.38, 0.36, 0.34, 0.31999999999999995, 0.29999999999999993, 0.28, 0.26, 0.24, 0.21999999999999997, 0.19999999999999996, 0.17999999999999994, 0.16000000000000003, 0.14, 0.12, 0.09999999999999998, 0.07999999999999996, 0.05999999999999995, 0.040000000000000036, 0.020000000000000018, -0.0]
  out "Plot X":dbl[](graph)=[0.0, 2e-08, 4e-08, 6e-08, 8e-08, 1e-07, 1.2e-07, 1.4e-07, 1.6e-07, 1.8e-07, 2e-07, 2.2e-07, 2.4e-07, 2.6e-07, 2.8e-07, 3e-07, 3.2e-07, 3.4e-07, 3.6e-07, 3.8e-07, 4e-07, 4.2e-07, 4.4e-07, 4.6e-07, 4.8e-07, 5e-07, 5.2e-07, 5.4e-07, 5.6e-07, 5.8e-07, 6e-07, 6.2e-07, 6.4e-07, 6.6e-07, 6.8e-07, 7e-07, 7.2e-07, 7.4e-07, 7.6e-07, 7.8e-07, 8e-07, 8.2e-07, 8.4e-07, 8.6e-07, 8.8e-07, 9e-07, 9.2e-07, 9.4e-07, 9.6e-07, 9.8e-07, 1e-06, 1.02e-06, 1.04e-06, 1.06e-06, 1.08e-06, 1.1e-06, 1.1199999999999999e-06, 1.1399999999999999e-06, 1.16e-06, 1.18e-06, 1.2e-06, 1.22e-06, 1.24e-06, 1.26e-06, 1.28e-06, 1.2999999999999998e-06, 1.32e-06, 1.3399999999999999e-06, 1.36e-06, 1.38e-06, 1.4e-06, 1.42e-06, 1.44e-06, 1.46e-06, 1.4799999999999998e-06, 1.5e-06, 1.5199999999999998e-06, 1.54e-06, 1.5599999999999999e-06, 1.58e-06, 1.6e-06, 1.62e-06, 1.64e-06, 1.66e-06, 1.68e-06, 1.6999999999999998e-06, 1.72e-06, 1.7399999999999999e-06, 1.76e-06, 1.78e-06, 1.8e-06, 1.82e-06, 1.84e-06, 1.86e-06, 1.88e-06, 1.9e-06, 1.92e-06, 1.94e-06, 1.96e-06, 1.9799999999999997e-06, 2e-06, 2.0199999999999997e-06, 2.04e-06, 2.0599999999999998e-06, 2.08e-06, 2.1e-06, 2.12e-06, 2.14e-06, 2.16e-06, 2.18e-06, 2.2e-06, 2.22e-06, 2.2399999999999997e-06, 2.26e-06, 2.2799999999999998e-06, 2.3e-06, 2.32e-06, 2.34e-06, 2.36e-06, 2.38e-06, 2.4e-06, 2.4199999999999997e-06, 2.44e-06, 2.4599999999999997e-06, 2.48e-06, 2.4999999999999998e-06, 2.52e-06, 2.54e-06, 2.56e-06, 2.58e-06, 2.5999999999999997e-06, 2.62e-06, 2.64e-06, 2.66e-06, 2.6799999999999998e-06, 2.7e-06, 2.72e-06, 2.74e-06, 2.76e-06, 2.78e-06, 2.8e-06, 2.82e-06, 2.84e-06, 2.8599999999999997e-06, 2.88e-06, 2.8999999999999998e-06, 2.92e-06, 2.94e-06, 2.9599999999999996e-06, 2.98e-06, 3e-06]
  out "x":dbl[](array[numeric])=[0.0, 2e-08, 4e-08, 6e-08, 8e-08, 1e-07, 1.2e-07, 1.4e-07, 1.6e-07, 1.8e-07, 2e-07, 2.2e-07, 2.4e-07, 2.6e-07, 2.8e-07, 3e-07, 3.2e-07, 3.4e-07, 3.6e-07, 3.8e-07, 4e-07, 4.2e-07, 4.4e-07, 4.6e-07, 4.8e-07, 5e-07, 5.2e-07, 5.4e-07, 5.6e-07, 5.8e-07, 6e-07, 6.2e-07, 6.4e-07, 6.6e-07, 6.8e-07, 7e-07, 7.2e-07, 7.4e-07, 7.6e-07, 7.8e-07, 8e-07, 8.2e-07, 8.4e-07, 8.6e-07, 8.8e-07, 9e-07, 9.2e-07, 9.4e-07, 9.6e-07, 9.8e-07, 1e-06, 1.02e-06, 1.04e-06, 1.06e-06, 1.08e-06, 1.1e-06, 1.1199999999999999e-06, 1.1399999999999999e-06, 1.16e-06, 1.18e-06, 1.2e-06, 1.22e-06, 1.24e-06, 1.26e-06, 1.28e-06, 1.2999999999999998e-06, 1.32e-06, 1.3399999999999999e-06, 1.36e-06, 1.38e-06, 1.4e-06, 1.42e-06, 1.44e-06, 1.46e-06, 1.4799999999999998e-06, 1.5e-06, 1.5199999999999998e-06, 1.54e-06, 1.5599999999999999e-06, 1.58e-06, 1.6e-06, 1.62e-06, 1.64e-06, 1.66e-06, 1.68e-06, 1.6999999999999998e-06, 1.72e-06, 1.7399999999999999e-06, 1.76e-06, 1.78e-06, 1.8e-06, 1.82e-06, 1.84e-06, 1.86e-06, 1.88e-06, 1.9e-06, 1.92e-06, 1.94e-06, 1.96e-06, 1.9799999999999997e-06, 2e-06, 2.0199999999999997e-06, 2.04e-06, 2.0599999999999998e-06, 2.08e-06, 2.1e-06, 2.12e-06, 2.14e-06, 2.16e-06, 2.18e-06, 2.2e-06, 2.22e-06, 2.2399999999999997e-06, 2.26e-06, 2.2799999999999998e-06, 2.3e-06, 2.32e-06, 2.34e-06, 2.36e-06, 2.38e-06, 2.4e-06, 2.4199999999999997e-06, 2.44e-06, 2.4599999999999997e-06, 2.48e-06, 2.4999999999999998e-06, 2.52e-06, 2.54e-06, 2.56e-06, 2.58e-06, 2.5999999999999997e-06, 2.62e-06, 2.64e-06, 2.66e-06, 2.6799999999999998e-06, 2.7e-06, 2.72e-06, 2.74e-06, 2.76e-06, 2.78e-06, 2.8e-06, 2.82e-06, 2.84e-06, 2.8599999999999997e-06, 2.88e-06, 2.8999999999999998e-06, 2.92e-06, 2.94e-06, 2.9599999999999996e-06, 2.98e-06, 3e-06]
  out "y":dbl[](array[numeric])=[0.0, 0.09580813208007743, 0.1824989149382628, 0.26093997906717925, 0.33191638900158116, 0.3961385005080873, 0.45424907006445175, 0.5068296877824316, 0.5544065981571044, 0.5974559668986514, 0.6364086465588308, 0.6716544886481295, 0.7035462454007136, 0.7324031002373527, 0.7585138622603756, 0.7821398567522392, 0.8035175406067887, 0.8228608688693284, 0.8403634360706267, 0.8562004137860504, 0.8705303038115675, 0.8834965245029955, 0.8952288461551118, 0.90584468978638, 0.9154503023279702, 0.9241418199787564, 0.932006230368708, 0.9391222431603269, 0.9455610778014061, 0.9513871763132007, 0.9566588482478362, 0.9614288542699043, 0.9657449342029285, 0.9696502848255628, 0.9731839921994724, 0.9763814228557754, 0.9792745777551737, 0.9818924125643232, 0.9842611274538788, 0.9864044293186076, 0.9883437690439604, 0.9900985561937433, 0.9916863532675555, 0.9931230514721888, 0.994423029766166, 0.9955992987691913, 0.9966636309768043, 0.9976266785834734, 0.9984980800933375, 0.9992865567855956, 1.0, 1.0, 1.0, 1.0, 1.0, 1.0, 1.0, 1.0, 1.0, 1.0, 1.0, 1.0, 1.0, 1.0, 1.0, 1.0, 1.0, 1.0, 1.0, 1.0, 1.0, 1.0, 1.0, 1.0, 1.0, 1.0, 1.0, 1.0, 1.0, 1.0, 1.0, 1.0, 1.0, 1.0, 1.0, 1.0, 1.0, 1.0, 1.0, 1.0, 1.0, 1.0, 1.0, 1.0, 1.0, 1.0, 1.0, 1.0, 1.0, 1.0, 1.0, 0.98, 0.96, 0.94, 0.92, 0.9, 0.88, 0.86, 0.84, 0.8200000000000001, 0.8, 0.78, 0.76, 0.74, 0.72, 0.7, 0.6799999999999999, 0.6599999999999999, 0.64, 0.62, 0.6, 0.5800000000000001, 0.56, 0.54, 0.52, 0.5, 0.48, 0.45999999999999996, 0.43999999999999995, 0.42000000000000004, 0.4, 0.38, 0.36, 0.33999999999999997, 0.31999999999999995, 0.29999999999999993, 0.28, 0.26, 0.24, 0.21999999999999997, 0.19999999999999996, 0.17999999999999994, 0.16000000000000003, 0.14, 0.12, 0.09999999999999998, 0.07999999999999996, 0.05999999999999994, 0.040000000000000036, 0.020000000000000018, 0.0]
  out "time for waveform":dbl[](array[numeric])=[0.0, 1e-06, 2e-06]
  out "timestep (ideal)":dbl[](array[numeric])=[1e-06, 2e-06, 3e-06]
  out "timestep":dbl[](array[numeric])=[50.0, 100.0, 150.0]
  out "timestep (int)":i32[](array[numeric])=[0, 50, 100]
  out "segment duration (int)":i32[](array[numeric])=[50, 50, 50]
  out "segment duration":dbl[](array[numeric])=[50.0, 50.0, 50.0]
  out "Plot Y":dbl[](graph)=[0.0, 0.09580813208007743, 0.1824989149382628, 0.26093997906717925, 0.33191638900158116, 0.3961385005080873, 0.45424907006445175, 0.5068296877824316, 0.5544065981571044, 0.5974559668986514, 0.6364086465588308, 0.6716544886481295, 0.7035462454007136, 0.7324031002373527, 0.7585138622603756, 0.7821398567522392, 0.8035175406067887, 0.8228608688693284, 0.8403634360706267, 0.8562004137860504, 0.8705303038115675, 0.8834965245029955, 0.8952288461551118, 0.90584468978638, 0.9154503023279702, 0.9241418199787564, 0.932006230368708, 0.9391222431603269, 0.9455610778014061, 0.9513871763132007, 0.9566588482478362, 0.9614288542699043, 0.9657449342029285, 0.9696502848255628, 0.9731839921994724, 0.9763814228557754, 0.9792745777551737, 0.9818924125643232, 0.9842611274538788, 0.9864044293186076, 0.9883437690439604, 0.9900985561937433, 0.9916863532675555, 0.9931230514721888, 0.994423029766166, 0.9955992987691913, 0.9966636309768043, 0.9976266785834734, 0.9984980800933375, 0.9992865567855956, 1.0, 1.0, 1.0, 1.0, 1.0, 1.0, 1.0, 1.0, 1.0, 1.0, 1.0, 1.0, 1.0, 1.0, 1.0, 1.0, 1.0, 1.0, 1.0, 1.0, 1.0, 1.0, 1.0, 1.0, 1.0, 1.0, 1.0, 1.0, 1.0, 1.0, 1.0, 1.0, 1.0, 1.0, 1.0, 1.0, 1.0, 1.0, 1.0, 1.0, 1.0, 1.0, 1.0, 1.0, 1.0, 1.0, 1.0, 1.0, 1.0, 1.0, 1.0, 0.98, 0.96, 0.94, 0.92, 0.9, 0.88, 0.86, 0.84, 0.8200000000000001, 0.8, 0.78, 0.76, 0.74, 0.72, 0.7, 0.6799999999999999, 0.6599999999999999, 0.64, 0.62, 0.6, 0.5800000000000001, 0.56, 0.54, 0.52, 0.5, 0.48, 0.45999999999999996, 0.43999999999999995, 0.42000000000000004, 0.4, 0.38, 0.36, 0.33999999999999997, 0.31999999999999995, 0.29999999999999993, 0.28, 0.26, 0.24, 0.21999999999999997, 0.19999999999999996, 0.17999999999999994, 0.16000000000000003, 0.14, 0.12, 0.09999999999999998, 0.07999999999999996, 0.05999999999999994, 0.040000000000000036, 0.020000000000000018, 0.0]
  # "Indicator"
  # "Commands that cause error:\n:SOUR1:DATA:COPY 000.RAF, VOLATILE\n:SOUR1:FUNC USER 000.RAF"
  # "Max 5 GSa/s"
  # "segment"
  # "segment name"
  # "repeat"
  # "jump flag"
  # "Resolution: 20ns, Range(Vint, Vfinal) is +/-1V\nIf e-factor =0 for exp rise/exp decay, will get NaN"
  # "Max 60 MSa/s\nfor arbitrary wf\nDefault: 50M"
  # "loss 5 % on a resistor"
  # "V initial"
  # "V final"
  # "Waveform"
  # "duration (us)"
  # "e-factor"
  # "Resolution: 20ns, Range(Vint, Vfinal) is +/-1V\nIf e-factor =0 for exp rise/exp decay, will get NaN"
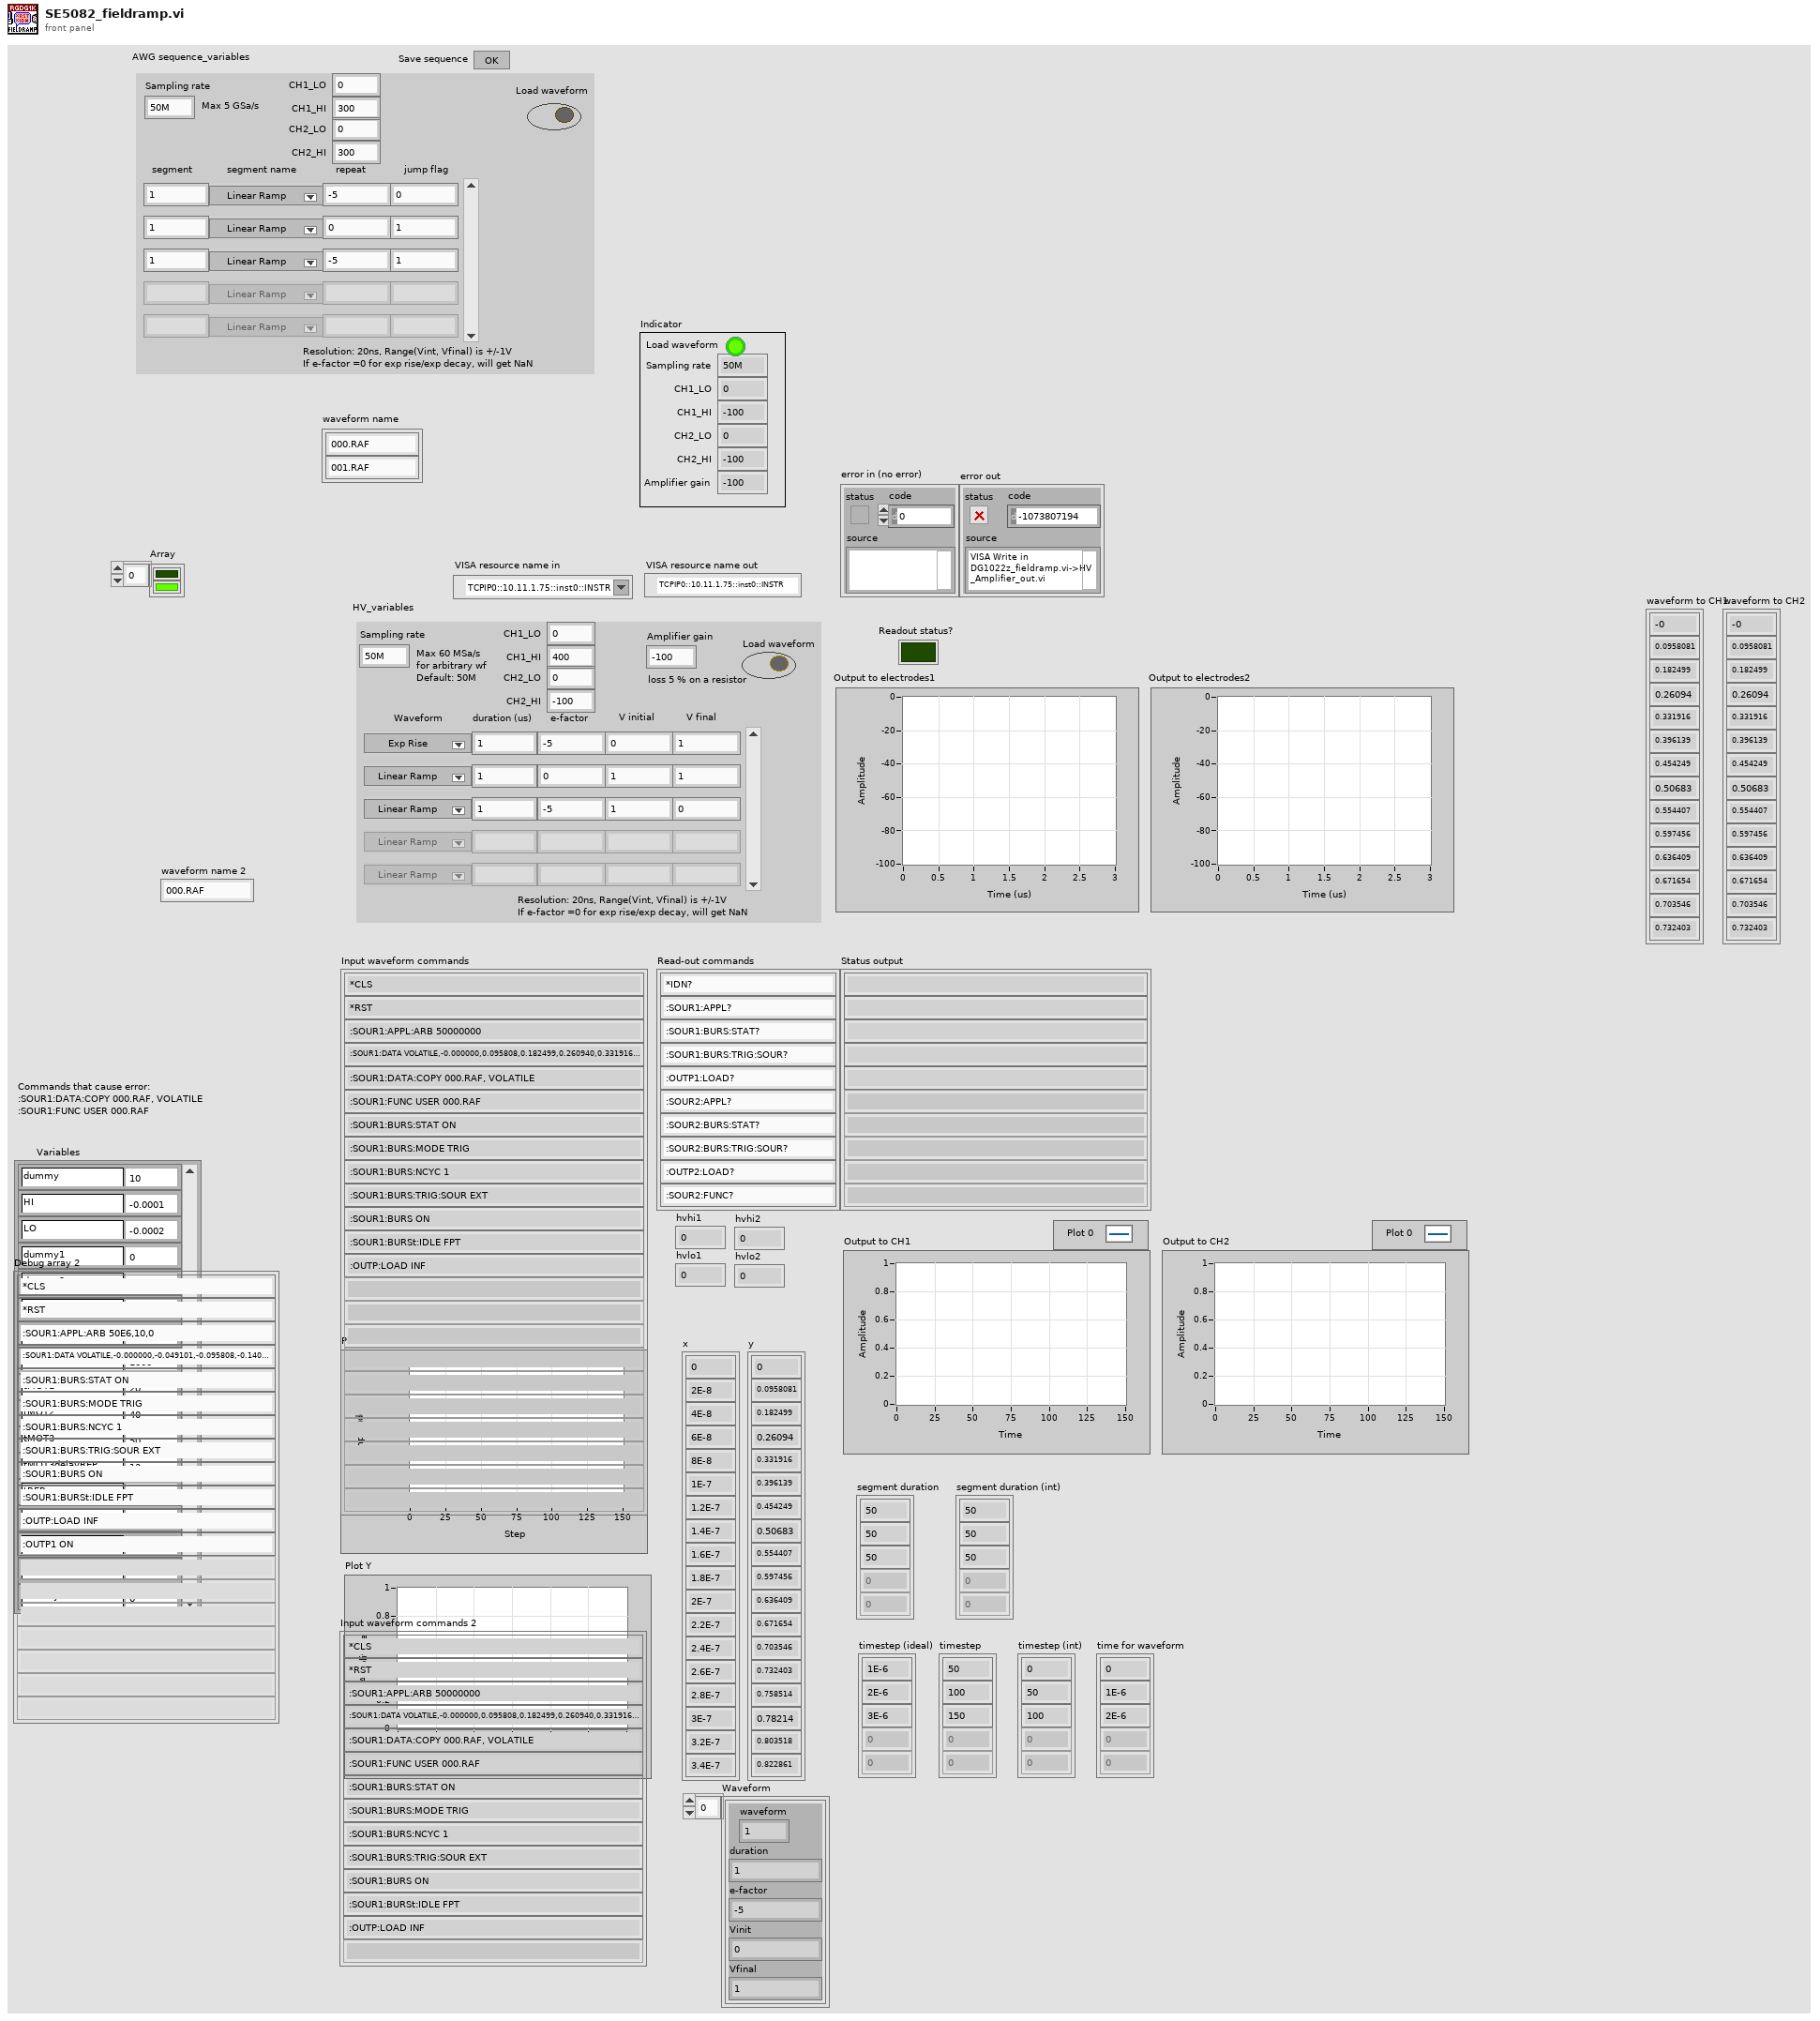
[diagram p1: front panel]
types:
  T1 = typedef "sequence_variables.ctl" = cluster{"Sampling rate":i32, "Waveform":cluster{"segment number":string, "repeat":string, "jump flag":string, "segment name":u16}[], "Load waveform":bool, "CH1_LO":string, "CH1_HI":string, "CH2_LO":string, "CH2_HI":string}
  T2 = cluster{"waveform":u16, "duration":string, "e-factor":string, "Vinit":string, "Vfinal":string}[]
  T3 = typedef "HV_variables.ctl" = cluster{"Sampling rate":i32, "Amplifier gain":dbl, "Waveform":cluster{"waveform":u16, "duration":string, "e-factor":string, "Vinit":string, "Vfinal":string}[], "Load waveform":bool, "CH1_LO":string, "CH1_HI":string, "CH2_LO":string, "CH2_HI":string}
  T4 = typedef "variables.ctl" = cluster{"Value":dbl, "Variable":string, "Save with Image":bool}[]
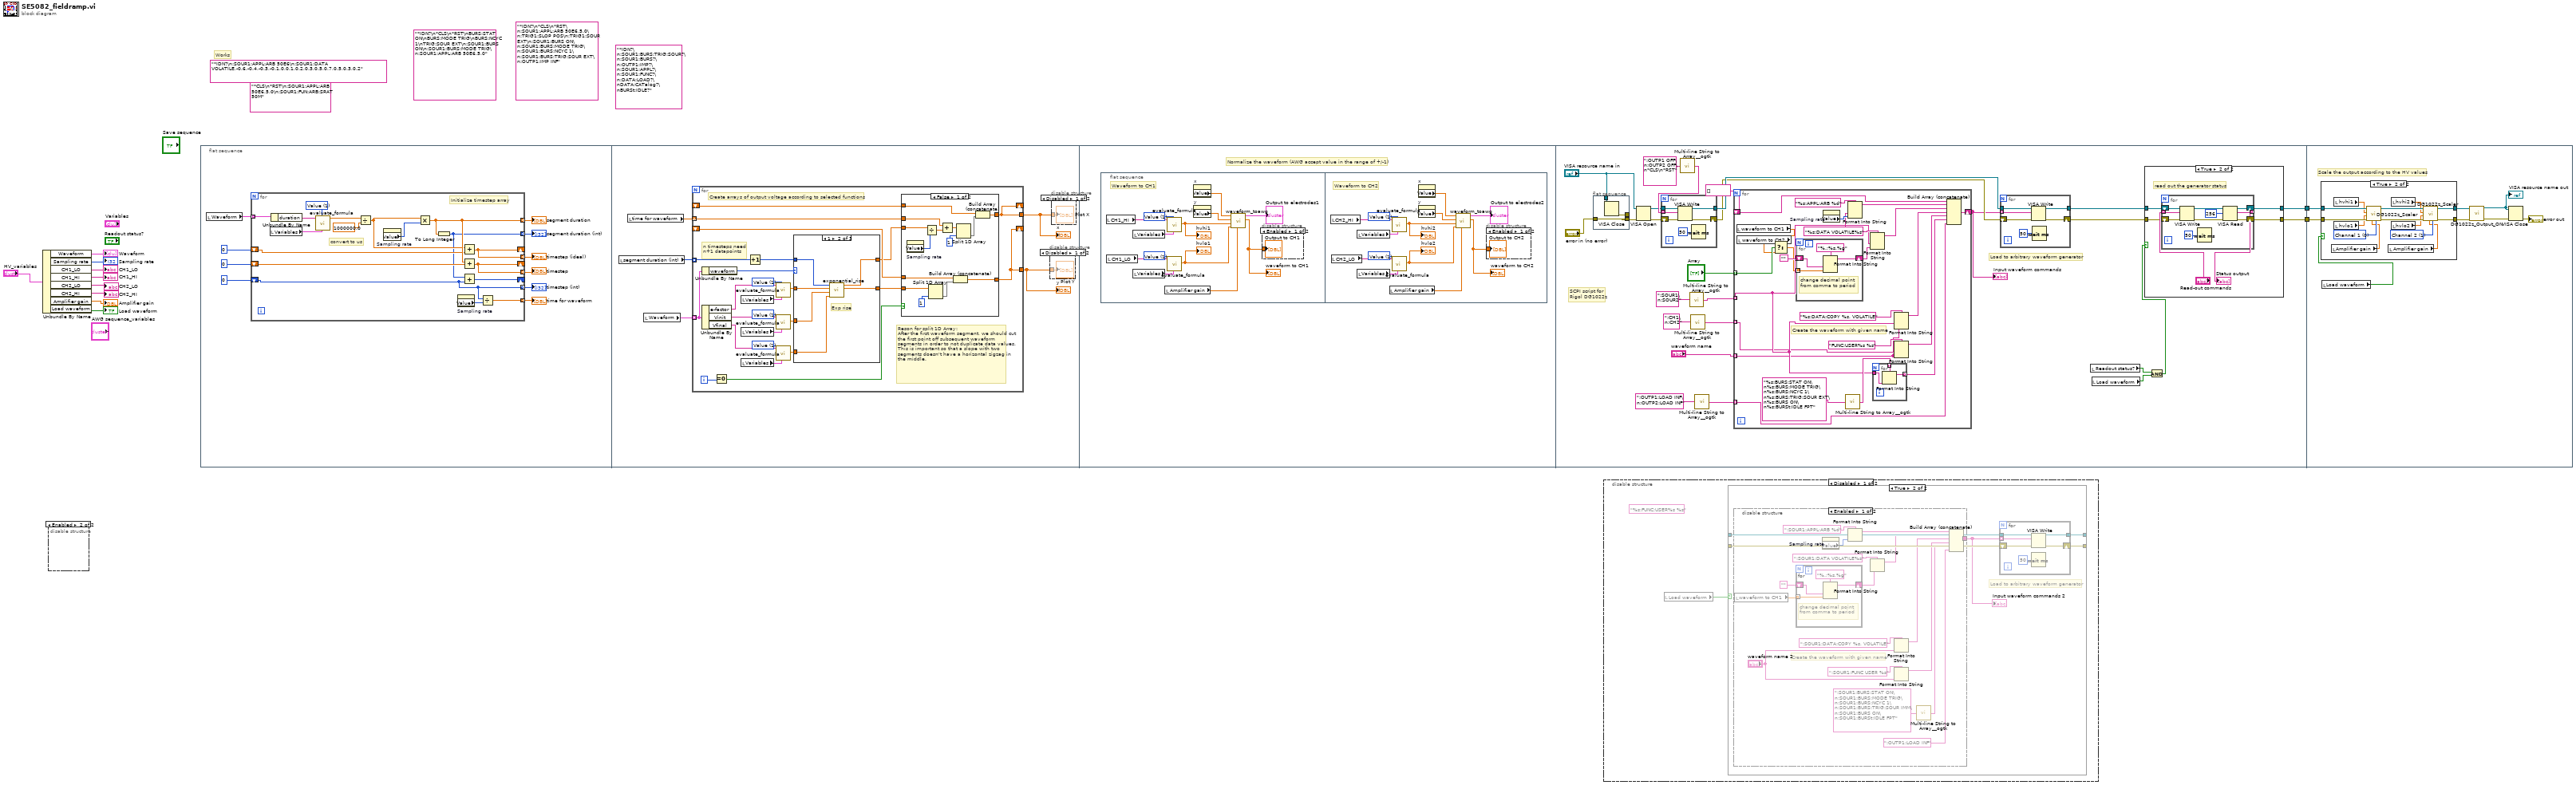
[diagram p0: block diagram]
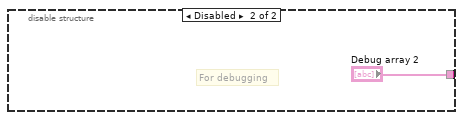
[diagram p3: hidden frame]
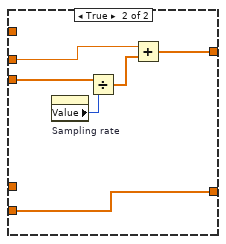
[diagram p7: hidden frame]
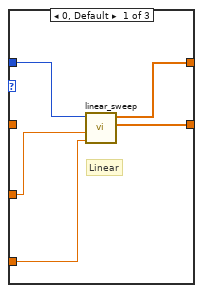
[diagram p8: hidden frame]
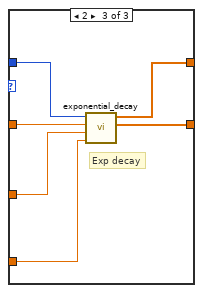
[diagram p9: hidden frame]
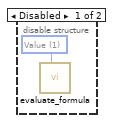
[diagram p14: hidden frame]
diagram:
  (unwired) "*IDN?\n:SOUR1:BURS:TRIG:SOUR?\n:SOUR1:BURS?\n:OUTP1:IMP?\n:SOUR1:APPL?\n:SOUR1:FUNC?\n:DATA:LOAD?\nDATA:CATalog?\nBURSt:IDLE?"
  (unwired) "*CLS\n*RST\n:SOUR1:APPL:ARB 50E6,5,0\n:SOUR1:FUN:ARB:SRAT 50M"
  (unwired) "*IDN?\n*CLS\n*RST\n:SOUR1:APPL:ARB 50E6,5,0\n:TRIG1:SLOP POS\n:TRIG1:SOUR EXT\n:SOUR1:BURS ON\n:SOUR1:BURS:MODE TRIG\n:SOUR1:BURS:NCYC 1\n:SOUR1:BURS:TRIG:SOUR EXT\n:OUTP1:IMP INF"
  (unwired) "*IDN?\n*CLS\n*RST\nBURS:STAT ON\nBURS:MODE TRIG\nBURS:NCYC 1\nTRIG:SOUR EXT\n:SOUR1:BURS ON\n:SOUR1:BURS:MODE TRIG\n:SOUR1:APPL:ARB 50E6,5,0"
  (unwired) "*IDN?\n:SOUR1:APPL:ARB 50E6\n:SOUR1:DATA VOLATILE,-0.6,-0.4,-0.3,-0.1,0,0.1,0.2,0.3,0.5,0.7,0.5,0.3,0.2"
  # "Works"
  n1 = Unbundle By Name("HV_variables") -> ("Waveform"=→"Waveform":T2, "Sampling rate"=→"Sampling rate":i32, "CH1_LO"=→"CH1_LO":string, "CH1_HI"=→"CH1_HI":string, "CH2_LO"=→"CH2_LO":string, "CH2_HI"=→"CH2_HI":string, "Amplifier gain"=→"Amplifier gain":dbl, "Load waveform"=→"Load waveform":bool)
  n2 = disable-structure shown="Enabled" {
    frame Disabled {
      w12 = u16 1 items=["Time in counts", "Value"] ("Time or Value")
      n3 = call "evaluate_formula.vi"("Time or Value"=w12) -> ()  [unwired: 9 in, 2 out]
    }
    frame Enabled {
    }
  }
  n4 = flat-sequence {
    tunnel: [w162] -> w5
    tunnel: [w161] -> w4
    tunnel: w5 -> [w235]
    tunnel: w4 -> [w234]
    frame #0 {
      n5 = local read "Waveform"() -> (w13:T2)
      n6 = for {
        tunnel: w13 -> [w40] mode=indexing
        tunnel: [w33] -> w22 mode=indexing
        tunnel: [w23] -> w21 mode=indexing
        shift-right: [w24] -> _
        shift-left: 0 -> [w25]
        tunnel: [w25] -> w19 mode=indexing
        shift-right: [w32] -> _
        shift-left: 0 -> [w34]
        tunnel: [w32] -> w17 mode=indexing
        shift-right: [w29] -> _
        shift-left: 0 -> [w31]
        tunnel: [w29] -> w15 mode=indexing
        tunnel: [w27] -> w14 mode=indexing
        w38 = u16 1 items=["Time in counts", "Value"] ("Time or Value")
        # "Initialize timestep array"
        # "convert to us"
        n7 = local read "Variables"() -> (w26:T4)
        n8 = Unbundle By Name(w40) -> ("duration"=w39:string)
        n9 = call "evaluate_formula.vi"("Variable array"=w26, "Time or Value"=w38, "Formula"=w39) -> ("Output"=w37:dbl)  [unwired: 7 in, 1 out]
        n10 = Divide(x=w37, y=1000000.0) -> (x/y=w30:dbl)
        n11 = property on="Sampling rate" class="DigNum (strict)"() -> ("Value"=w35:i32)  [unwired: 2 in, 2 out]
        n12 = Multiply(x=w30, y=w35) -> (x*y=w33:dbl)
        n13 = To Long Integer(number=w33) -> (32bit integer=w23:i32)
        n14 = property on="Sampling rate" class="DigNum (strict)"() -> ("Value"=w28:i32)  [unwired: 2 in, 2 out]
        n15 = Add(x=w30, y=w31) -> (x+y=w29:dbl)
        n16 = Add(x=w33, y=w34) -> (x+y=w32:dbl)
        n17 = Add(x=w23, y=w25) -> (x+y=w24:i32)
        n18 = Divide(x=w25, y=w28) -> (x/y=w27:dbl)
      }
      "segment duration" <- w22
      "segment duration (int)" <- w21
      "timestep (int)" <- w19
      "timestep" <- w17
      "timestep (ideal)" <- w15
      "time for waveform" <- w14
    }
    frame #1 {
      n19 = local read "segment duration (int)"() -> (w45:i32[])
      n20 = local read "time for waveform"() -> (w43:dbl[])
      n21 = local read "Waveform"() -> (w44:T2)
      n22 = for {
        tunnel: w44 -> [w70] mode=indexing
        tunnel: w45 -> [w69] mode=indexing
        shift-right: [w66] -> _
        shift-left: _ -> [w67]
        tunnel: [w66] -> w41
        shift-right: [w51] -> _
        shift-left: _ -> [w52]
        tunnel: [w51] -> w42
        tunnel: w43 -> [w49] mode=indexing
        i -> [w68]
        w61 = u16 1 items=["Time in counts", "Value"] ("Time or Value")
        w62 = u16 1 items=["Time in counts", "Value"] ("Time or Value")
        w65 = u16 1 items=["Time in counts", "Value"] ("Time or Value")
        # "Create arrays of output voltage according to selected functions"
        # "Reson for split 1D Array:\nAfter the first waveform segment, we should cut the first point off subsequent waveform segments in order to not duplicate data values. This is important so that a slope with two segments doesn't have a horizontal zigzag in the middle."
        # "n timesteps need n+1 datapoints"
        n23 = Unbundle By Name(w70) -> ("waveform"=w72:u16)
        n24 = Unbundle By Name(w70) -> ("e-factor"=w57:string, "Vinit"=w59:string, "Vfinal"=w58:string)
        n25 = Equal To 0?(x=w68) -> (x = 0?=w48:bool)
        n26 = local read "Variables"() -> (w60:T4)
        n27 = local read "Variables"() -> (w63:T4)
        n28 = local read "Variables"() -> (w64:T4)
        n29 = Increment(x=w69) -> (x+1=w50:i32)
        n30 = call "evaluate_formula.vi"("Variable array"=w60, "Time or Value"=w61, "Formula"=w57) -> ("Output"=w56:dbl)  [unwired: 7 in, 1 out]
        n31 = call "evaluate_formula.vi"("Variable array"=w63, "Time or Value"=w62, "Formula"=w59) -> ("Output"=w55:dbl)  [unwired: 7 in, 1 out]
        n32 = call "evaluate_formula.vi"("Variable array"=w64, "Time or Value"=w65, "Formula"=w58) -> ("Output"=w54:dbl)  [unwired: 7 in, 1 out]
        n33 = case shown="1" w72 {
          tunnel: w50 -> [w97 w103 w109]
          tunnel: w56 -> [_ w102 w108]
          tunnel: [w96 w101 w107] -> w71
          tunnel: w55 -> [w94 w99 w105]
          tunnel: w54 -> [w95 w100 w106]
          tunnel: [w93 w98 w104] -> w53
          frame 0, Default {
            # "Linear"
            n34 = call "linear_sweep.vi"("yf"=w95, "yi"=w94, "number of x points"=w97) -> ("y"=w96:dbl[], "x"=w93:dbl[])  [unwired: 7 in]
          }
          frame 1 {
            # "Exp rise"
            n35 = call "exponential_rise.vi"("yf"=w100, "yi"=w99, "e-factor"=w102, "number of x points"=w103) -> ("y"=w101:dbl[], "x"=w98:dbl[])  [unwired: 6 in]
          }
          frame 2 {
            # "Exp decay"
            n36 = call "exponential_decay.vi"("yf"=w106, "yi"=w105, "e-factor"=w108, "number of x points"=w109) -> ("y"=w107:dbl[], "x"=w104:dbl[])  [unwired: 6 in]
          }
        }
        n37 = case shown="False" w48 {
          tunnel: w71 -> [w79 w92]
          tunnel: [w83 w92] -> w66
          tunnel: w67 -> [w84 _]
          tunnel: w53 -> [w74 w91]
          tunnel: [w81 w87] -> w51
          tunnel: w52 -> [w82 _]
          tunnel: w49 -> [w75 w89]
          frame False {
            n38 = property on="Sampling rate" class="DigNum (strict)"() -> ("Value"=w77:i32)  [unwired: 2 in, 2 out]
            n39 = Divide(x=w74, y=w77) -> (x/y=w76:dbl[])
            n40 = Split 1D Array(array=w79, index=1) -> (second subarray=w78:dbl[])  [unwired: 1 out]
            n41 = Add(x=w75, y=w76) -> (x+y=w73:dbl[])
            n42 = Build Array (concatenate)(w84, w78) -> (w83:dbl[])
            n43 = Split 1D Array(array=w73, index=1) -> (second subarray=w80:dbl[])  [unwired: 1 out]
            n44 = Build Array (concatenate)(w82, w80) -> (w81:dbl[])
          }
          frame True {
            n45 = property on="Sampling rate" class="DigNum (strict)"() -> ("Value"=w90:i32)  [unwired: 2 in, 2 out]
            n46 = Divide(x=w91, y=w90) -> (x/y=w88:dbl[])
            n47 = Add(x=w89, y=w88) -> (x+y=w87:dbl[])
          }
        }
      }
      "y" <- w41
      "x" <- w42
      n48 = disable-structure shown="Disabled" {
        disable-tunnel: w41 -> [w47 _]
        frame Disabled {
          "Plot Y" <- w47
        }
        frame Enabled {
        }
      }
      n49 = disable-structure shown="Disabled" {
        disable-tunnel: w42 -> [w46 _]
        frame Disabled {
          "Plot X" <- w46
        }
        frame Enabled {
        }
      }
    }
    frame #2 {
      # "Normalize the waveform (AWG accept value in the range of +/-1)"
      n50 = flat-sequence {
        frame #0 {
          w119 = u16 1 items=["Time in counts", "Value"] ("Time or Value")
          w122 = u16 1 items=["Time in counts", "Value"] ("Time or Value")
          # "Waveform to CH1"
          n51 = local read "CH1_HI"() -> (w116:string)
          n52 = local read "CH1_LO"() -> (w115:string)
          n53 = local read "Variables"() -> (w121:T4)
          n54 = local read "Variables"() -> (w120:T4)
          n55 = local read "Amplifier gain"() -> (w110:dbl)
          n56 = call "evaluate_formula.vi"("Variable array"=w121, "Time or Value"=w122, "Formula"=w116) -> ("Output"=w118:dbl)  [unwired: 7 in, 1 out]
          "hvhi1" <- w118
          n57 = call "evaluate_formula.vi"("Variable array"=w120, "Time or Value"=w119, "Formula"=w115) -> ("Output"=w117:dbl)  [unwired: 7 in, 1 out]
          "hvlo1" <- w117
          n58 = property on="x" class="Arr (strict)"() -> ("Value"=w112:dbl[])  [unwired: 2 in, 2 out]
          n59 = property on="y" class="Arr (strict)"() -> ("Value"=w111:dbl[])  [unwired: 2 in, 2 out]
          n60 = call "waveform_toawg.vi"("Amplifier gain"=w110, "HV_LO"=w117, "HV_HI"=w118, "y"=w111, "x"=w112) -> ("waveform to awg"=w113:dbl[], "Output to electrodes"=→"Output to electrodes1":cluster{dbl[], "y":dbl[]})  [unwired: 5 in]
          "waveform to CH1" <- w113
          n61 = disable-structure shown="Enabled" {
            disable-tunnel: w113 -> [w123 _]
            frame Enabled {
              "Output to CH1" <- w123
            }
            frame Disabled {
            }
          }
        }
        frame #1 {
          w127 = u16 1 items=["Time in counts", "Value"] ("Time or Value")
          w124 = u16 1 items=["Time in counts", "Value"] ("Time or Value")
          # "Waveform to CH2"
          n62 = local read "CH2_HI"() -> (w130:string)
          n63 = local read "CH2_LO"() -> (w131:string)
          n64 = local read "Variables"() -> (w125:T4)
          n65 = local read "Variables"() -> (w126:T4)
          n66 = local read "Amplifier gain"() -> (w136:dbl)
          n67 = call "evaluate_formula.vi"("Variable array"=w125, "Time or Value"=w124, "Formula"=w130) -> ("Output"=w128:dbl)  [unwired: 7 in, 1 out]
          "hvhi2" <- w128
          n68 = call "evaluate_formula.vi"("Variable array"=w126, "Time or Value"=w127, "Formula"=w131) -> ("Output"=w129:dbl)  [unwired: 7 in, 1 out]
          "hvlo2" <- w129
          n69 = property on="x" class="Arr (strict)"() -> ("Value"=w134:dbl[])  [unwired: 2 in, 2 out]
          n70 = property on="y" class="Arr (strict)"() -> ("Value"=w135:dbl[])  [unwired: 2 in, 2 out]
          n71 = call "waveform_toawg.vi"("Amplifier gain"=w136, "HV_LO"=w129, "HV_HI"=w128, "y"=w135, "x"=w134) -> ("waveform to awg"=w133:dbl[], "Output to electrodes"=→"Output to electrodes2":cluster{dbl[], "y":dbl[]})  [unwired: 5 in]
          "waveform to CH2" <- w133
          n72 = disable-structure shown="Enabled" {
            disable-tunnel: w133 -> [w137 _]
            frame Enabled {
              "Output to CH2" <- w137
            }
            frame Disabled {
            }
          }
        }
      }
    }
    frame #3 {
      # "Load to arbitrary waveform generator"
      # "SCPI script for\nRigol DG1022z"
      n73 = flat-sequence {
        tunnel: "VISA resource name in" -> [w209]
        tunnel: "error in (no error)" -> [w208]
        tunnel: [w208] -> w157
        tunnel: [w207] -> _
        frame #0 {
          n74 = VISA Close(VISA resource name=w209) -> (error out=w207:errorcluster)  [unwired: 1 in]
        }
      }
      n75 = VISA Open(error in (no error)=w157, VISA resource name="VISA resource name in") -> (VISA resource name=w154:refnum<visa-resource-name>, error out=w153:errorcluster)  [unwired: 3 in]
      n76 = call <userlib>:"Multi-line String to Array__ogtk.vi"("string"=":OUTP1 OFF\n:OUTP2 OFF\n*CLS\n*RST") -> ("lines"=w155:string[])
      n77 = for {
        tunnel: w154 -> [w206]
        tunnel: w155 -> [w205] mode=indexing
        shift-right: [w203] -> w151
        shift-left: w153 -> [w204]
        tunnel: [w202] -> w152
        n78 = VISA Write(VISA resource name=w206, write buffer=w205, error in (no error)=w204) -> (VISA resource name out=w202:refnum<visa-resource-name>, error out=w203:errorcluster)  [unwired: 1 out]
        n79 = Wait (ms)(milliseconds to wait=u32 50) -> ()  [unwired: 1 out]
      }
      n80 = call <userlib>:"Multi-line String to Array__ogtk.vi"("string"=":SOUR1\n:SOUR2" ("format string")) -> ("lines"=w143:string[])
      n81 = call <userlib>:"Multi-line String to Array__ogtk.vi"("string"=":CH1\n:CH2" ("format string")) -> ("lines"=w139:string[])
      n82 = call <userlib>:"Multi-line String to Array__ogtk.vi"("string"=":OUTP1:LOAD INF\n:OUTP2:LOAD INF" ("element")) -> ("lines"=w141:string[])
      n83 = for {
        tunnel: w143 -> [w170] mode=indexing
        tunnel: "waveform name" -> [w164] mode=indexing
        shift-right: [w174] -> w147
        shift-left: string[] [] -> [w175]
        tunnel: w141 -> [w171] mode=indexing
        tunnel: w139 -> [w165] mode=indexing
        tunnel: "Array" -> [w169] mode=indexing
        # "Create the waveform with given name"
        n84 = local read "waveform to CH1"() -> (w166:dbl[])
        n85 = local read "waveform to CH2"() -> (w167:dbl[])
        n86 = Select(t=w166, s=w169, f=w167) -> (s? t:f=w168:dbl[])
        n87 = for {
          tunnel: w168 -> [w193] mode=indexing
          shift-right: [w192] -> w176
          shift-left: "" -> [w191]
          # "change decimal point from comma to period"
          n88 = Format Into String(format string="%.;%s,%g", w191, w193) -> (resulting string=w192:string)  [unwired: 2 in, 1 out]
        }
        n89 = property on="Sampling rate" class="DigNum (strict)"() -> ("Value"=w177:i32)  [unwired: 2 in, 2 out]
        n90 = call <userlib>:"Multi-line String to Array__ogtk.vi"("string"="%s:BURS:STAT ON\n%s:BURS:MODE TRIG\n%s:BURS:NCYC 1\n%s:BURS:TRIG:SOUR EXT\n%s:BURS ON\n%s:BURSt:IDLE FPT" ("element")) -> ("lines"=w173:string[])
        n91 = Format Into String(format string="%s:APPL:ARB %d", w170, w177) -> (resulting string=w181:string)  [unwired: 2 in, 1 out]
        n92 = Format Into String(format string="%s:DATA VOLATILE%s" ("string"), w170, w176) -> (resulting string=w184:string)  [unwired: 2 in, 1 out]
        n93 = for {
          tunnel: w170 -> [w190]
          tunnel: w173 -> [w189] mode=indexing
          tunnel: [w188] -> w172 mode=indexing
          n94 = Format Into String(format string=w189, w190) -> (resulting string=w188:string)  [unwired: 2 in, 1 out]
        }
        n95 = Format Into String(format string="%s:DATA:COPY %s, VOLATILE", w170, w164) -> (resulting string=w183:string)  [unwired: 2 in, 1 out]
        n96 = Format Into String(format string="FUNC:USER%s %s", w165, w164) -> (resulting string=w187:string)  [unwired: 2 in, 1 out]
        n97 = Build Array (concatenate)(w175, w181, w184, w183, w187, w172, w171) -> (w174:string[])
      }
      "Input waveform commands" <- w147
      n98 = for {
        tunnel: w152 -> [w200]
        tunnel: w147 -> [w199] mode=indexing
        shift-right: [w197] -> w163
        shift-left: w151 -> [w198]
        tunnel: [w196] -> w160
        n99 = VISA Write(VISA resource name=w200, write buffer=w199, error in (no error)=w198) -> (VISA resource name out=w196:refnum<visa-resource-name>, error out=w197:errorcluster)  [unwired: 1 out]
        n100 = Wait (ms)(milliseconds to wait=u32 50) -> ()  [unwired: 1 out]
      }
      n101 = local read "Readout status?"() -> (w149:bool)
      n102 = local read "Load waveform"() -> (w150:bool)
      n103 = And(x=w149, y=w150) -> (x .and. y?=w148:bool)
      n104 = case shown="True" w148 {
        tunnel: w160 -> [w211 w215]
        tunnel: w163 -> [w210 w214]
        tunnel: [w210 w213] -> w161
        tunnel: [w211 w212] -> w162
        frame False {
        }
        frame True {
          # "read out the generator status"
          n105 = for {
            tunnel: [w225] -> w217 mode=indexing
            shift-right: [w224] -> w213
            shift-left: w214 -> [w221]
            tunnel: "Read-out commands" -> [w222] mode=indexing
            shift-right: [w218] -> w212
            shift-left: w215 -> [w223]
            n106 = VISA Write(VISA resource name=w223, write buffer=w222, error in (no error)=w221) -> (VISA resource name out=w219:refnum<visa-resource-name>, error out=w226:errorcluster)  [unwired: 1 out]
            n107 = Wait (ms)(milliseconds to wait=u32 50) -> ()  [unwired: 1 out]
            n108 = VISA Read(VISA resource name=w219, byte count=u32 256, error in (no error)=w226) -> (VISA resource name out=w218:refnum<visa-resource-name>, read buffer=w225:string, error out=w224:errorcluster)  [unwired: 1 out]
          }
          "Status output" <- w217
        }
      }
    }
    frame #4 {
      # "Scale the output according to the HV values"
      n109 = local read "Load waveform"() -> (w233:bool)
      n110 = case shown="True" w233 {
        tunnel: w235 -> [w237 w251]
        tunnel: w234 -> [w236 w250]
        tunnel: [w237 w247] -> w231
        tunnel: [w236 w246] -> w230
        frame False {
        }
        frame True {
          w239 = u16 1 items=["Channel 1", "Channel 2"] ("Channel")
          w243 = u16 0 items=["Channel 1", "Channel 2"] ("Channel")
          n111 = local read "Amplifier gain"() -> (w242:dbl)
          n112 = local read "hvhi1"() -> (w245:dbl)
          n113 = local read "hvlo1"() -> (w244:dbl)
          n114 = call "DG1022z_Scaler.vi"("Channel"=w243, "Amplifier gain"=w242, "error in"=w250, "hvlo"=w244, "hvhi"=w245, "VISA resource name in"=w251) -> ("error out"=w249:errorcluster, "VISA resource name out"=w248:refnum<visa-resource-name>)  [unwired: 4 in]
          n115 = local read "Amplifier gain"() -> (w238:dbl)
          n116 = local read "hvhi2"() -> (w241:dbl)
          n117 = local read "hvlo2"() -> (w240:dbl)
          n118 = call "DG1022z_Scaler.vi"("Channel"=w239, "Amplifier gain"=w238, "error in"=w249, "hvlo"=w240, "hvhi"=w241, "VISA resource name in"=w248) -> ("error out"=w246:errorcluster, "VISA resource name out"=w247:refnum<visa-resource-name>)  [unwired: 4 in]
        }
      }
      n119 = call "DG1022z_Output_ON.vi"("error in"=w230, "VISA resource name in"=w231) -> ("error out"=w228:errorcluster, "VISA resource name out"=w229:refnum<visa-resource-name>)  [unwired: 8 in]
      "VISA resource name out" <- w229
      n120 = VISA Close(VISA resource name=w229, error in (no error)=w228) -> (error out=→"error out":errorcluster)
    }
  }
  n121 = disable-structure shown="Disabled" {
    frame Disabled {
      (unwired) "%s:FUNC:USER%s %s"
      n122 = local read "Load waveform"() -> (w252:bool)
      n123 = case shown="True" w252 {
        tunnel: [w253 w259] -> _
        tunnel: [w254 w258] -> _
        tunnel: _ -> [w253 w257]
        tunnel: _ -> [w254 w256]
        frame False {
        }
        frame True {
          # "Load to arbitrary waveform generator"
          n124 = disable-structure shown="Enabled" {
            disable-tunnel: [w268 "Debug array 2"] -> w255
            frame Enabled {
              # "Create the waveform with given name"
              n125 = local read "waveform to CH1"() -> (w272:dbl[])
              n126 = for {
                tunnel: w272 -> [w279] mode=indexing
                shift-right: [w278] -> w275
                shift-left: "" -> [w277]
                # "change decimal point from comma to period"
                n127 = Format Into String(format string="%.;%s,%g", w277, w279) -> (resulting string=w278:string)  [unwired: 2 in, 1 out]
              }
              n128 = property on="Sampling rate" class="DigNum (strict)"() -> ("Value"=w263:i32)  [unwired: 2 in, 2 out]
              n129 = Format Into String(format string=":SOUR1:APPL:ARB %d", w263) -> (resulting string=w266:string)  [unwired: 2 in, 1 out]
              n130 = Format Into String(format string=":SOUR1:DATA VOLATILE%s" ("string"), w275) -> (resulting string=w271:string)  [unwired: 2 in, 1 out]
              n131 = Format Into String(format string=":SOUR1:DATA:COPY %s, VOLATILE", "waveform name 2") -> (resulting string=w270:string)  [unwired: 2 in, 1 out]
              n132 = Format Into String(format string=":SOUR1:FUNC USER %s", "waveform name 2") -> (resulting string=w276:string)  [unwired: 2 in, 1 out]
              n133 = call <userlib>:"Multi-line String to Array__ogtk.vi"("string"=":SOUR1:BURS:STAT ON\n:SOUR1:BURS:MODE TRIG\n:SOUR1:BURS:NCYC 1\n:SOUR1:BURS:TRIG:SOUR IMM\n:SOUR1:BURS ON\n:SOUR1:BURSt:IDLE FPT" ("element")) -> ("lines"=w264:string[])
              n134 = Build Array (concatenate)(w266, w271, w270, w276, w264, ":OUTP1:LOAD INF" ("element")) -> (w268:string[])
            }
            frame Disabled {
              # "For debugging"
            }
          }
          "Input waveform commands 2" <- w255
          n135 = for {
            tunnel: w257 -> [w287]
            tunnel: w255 -> [w286] mode=indexing
            shift-right: [w284] -> w258
            shift-left: w256 -> [w285]
            tunnel: [w283] -> w259
            n136 = VISA Write(VISA resource name=w287, write buffer=w286, error in (no error)=w285) -> (VISA resource name out=w283:refnum<visa-resource-name>, error out=w284:errorcluster)  [unwired: 1 out]
            n137 = Wait (ms)(milliseconds to wait=u32 50) -> ()  [unwired: 1 out]
          }
        }
      }
    }
    frame Enabled {
    }
  }
